vi "EXO RealTime Controls.vi"() -> ()   [LabVIEW 2010]
uses:
  <vilib>/addons/control/pid/pid.llb/PID (DBL).vi
  <vilib>/Utility/error.llb/DialogType.ctl
  <vilib>/Instr/_visa.llb/VISA Configure Serial Port (Instr).vi
  <vilib>/Platform/TimedLoop/XDataNode/XDataNode.xnode
  <vilib>/Platform/TimedLoop/XDataNode/nitl_modes.ctl
  <vilib>/Platform/TimedLoop/XDataNode/XDNodeRunTimeDep.lvlib
  <vilib>/Platform/TimedLoop/XDataNode/wakeup.ctl
  <vilib>/Platform/TimedLoop/XDataNode/timing_clust.ctl
  <vilib>/FieldPoint/Polymorphic Read.llb/FP Read (Boolean -IO).vi
  <vilib>/Utility/file.llb/Write To Spreadsheet File (I64).vi
panel:
  in  "Start Yoyo":bool
  in  "Low dP limit for Yoyo":dbl=-100.0
  in  "High dP limit for Yoyo":dbl=100.0
  in  "Yoyo method while in\nAutomatic?":bool=TRUE
  in  "Yoyo\nMethod\nProp. Valves\nSetting":dbl(slide)=0.04 min=0.0 max=0.075 scale=0.0..0.075
  in  "Automatic Bleed\nWhen in Manual?":bool
  in  "Run All Fridges?":bool
  out "Actual dP Offset (torr)":dbl=100.0
  in  "dP Offset 2 (torr)":dbl
  in  "dP Offset 1 (torr)":dbl
  in  "Bleed 50?":bool
  in  "VX52 real":bool
  in  "Control TC":u16(ring)=37 items=["1", "2", "3", "4", "5", "6", "7", "8", "10", "11", "12", "13", "14", "15", "16", "17", "18", "19", "20", "21", "22", "23", "24", "25", "26", "27", "28", "29", "30", "31", "32", "33", "34", "35", "36", "37", "38", "39", "40"]
  in  "Enter Liquid\nLevel Manually?":bool
  in  "Manual Liquid\nLevel (cm)":dbl
  in  "HFE head disable":bool
  in  "Valves to Open":i32[](array[numeric])=[49, 51, 52, 0, 0, 0]
  out "Actual Pressure\n(psi)":dbl=20.47422134532471
  in  "Cryostat High Liquid\nLevel Alarm (cm)":dbl=300.0 min=0.0
  in  "Cryostat Low Liquid\nLevel Alarm (cm)":dbl=20.0
  in  "Ballast Bottle Low\nLevel Alarm (cm)":dbl min=0.0
  in  "Xenon Heater\nIn Use?":bool
  in  "Ring":u16(ring) items=["Normal Operation", "Vapour Fill Mode", "Pumpout Mode"]
  in  "baud rate 4":u32=9600
  in  "VISA resource name 4":refnum<visa-resource-name>="COM2"
  in  "data bits 4":u16=8 min=5 max=8 step=1
  in  "parity 4":u16(ring) items=["None", "Odd", "Even", "Mark", "Space"]
  in  "stop bits 4":u16(ring)=10 items=["1.0"=10, "1.5"=15, "2.0"=20]
  in  "flow control 4":u16(ring) items=["None"=0, "XON/XOFF"=1, "RTS/CTS"=2, "DTR/DSR"=4]
  in  "Prop Valve\nMult. Factor":dbl=0.04
  in  "V-X9":dbl(slide)=0.042 min=0.0 max=0.075 scale=0.0..0.075
  in  "V-X8":dbl(slide)=0.035 min=0.0 max=0.075 scale=0.0..0.075
  in  "V-X52":bool
  in  "V-X51":bool
  in  "V-X50":bool
  in  "V-X49":bool
  in  "V-X11":bool
  in  "V-X10":bool
  in  "Manual Operation of Valves":bool=TRUE
  in  "Restart all 3 Fridges until setpoint":bool
  in  "baud rate 3":u32=9600
  in  "VISA resource name 3":refnum<visa-resource-name>="COM2"
  in  "data bits 3":u16=8 min=5 max=8 step=1
  in  "parity 3":u16(ring) items=["None", "Odd", "Even", "Mark", "Space"]
  in  "stop bits 3":u16(ring)=10 items=["1.0"=10, "1.5"=15, "2.0"=20]
  in  "flow control 3":u16(ring) items=["None"=0, "XON/XOFF"=1, "RTS/CTS"=2, "DTR/DSR"=4]
  in  "baud rate 2":u32=9600
  in  "VISA resource name 2":refnum<visa-resource-name>="COM3"
  in  "data bits 2":u16=8 min=5 max=8 step=1
  in  "parity 2":u16(ring) items=["None", "Odd", "Even", "Mark", "Space"]
  in  "stop bits 2":u16(ring)=10 items=["1.0"=10, "1.5"=15, "2.0"=20]
  in  "flow control 2":u16(ring) items=["None"=0, "XON/XOFF"=1, "RTS/CTS"=2, "DTR/DSR"=4]
  in  "Condenser \nin Use?":bool=TRUE
  in  "HFE Relief to\nAtmosphere\nThreshold (torr)":dbl=1450.0 min=0.0
  in  "HFE Vapor Fill\nSet Point (torr)":dbl=890.0
  in  "Vapor Fill\nValve \n(HEV17)":bool
  in  "Relief To \nWessington\n(HEV28/18)":bool
  in  "HFE Relief to\nWessington \nThreshold (torr)":dbl=1350.0 min=0.0
  in  "Manual Operation of HFE Valves?":bool
  in  "Ballast Bottle \nHeater in use?":bool=TRUE
  out "Cryostat \nTemp. (K)":dbl=170.03219604492188
  out "Actual":dbl=999.1363027125445
  out "Actual":dbl=167.0546875
  in  "Valve 2 State":bool=TRUE
  in  "Valve 1 State":bool=TRUE
  in  "Manual Operation of Valves":bool
  in  "Heaters In Use?":bool
  in  "Heater Temperature\nHigh Cutoff Limit (K)":dbl=400.0 format="%.2f"
  in  "Cryostat Heater PID Gains":T1={"Proportional gain (Kc)"=1.0, "Integral time (Ti, min)"=0.01, "Derivative time (Td, min)"=0.0} {"Derivative time (Td, min)" format="%.3f"; "Integral time (Ti, min)" format="%.3f"; "Proportional gain (Kc)" format="%.3f"}
  in  "Reinitialize\nHeater PID":bool
  in  "Heater Output \nHigh Limit (Volts)":dbl min=0.0
  in  "Heater Output \nLow Limit (Volts)":dbl min=0.0
  in  "Temperature\nSet Point (K)":dbl=300.0 format="%.2f"
  in  "Folder to Store Data if Monitoring Program fails":string="c:/data/"
  in  "CC Shut-Off\nThreshold (Torr)":dbl=1.0
  in  "CC Soft Threshold\nAlarm (Torr)":dbl=1.0
  in  "TC 1/2 Shut-Off\nThreshold (Torr)":dbl=1.0
  in  "TC 1/2 Soft Threshold\nAlarm (Torr)":dbl=0.05
  in  "flow control":u16(ring) items=["None"=0, "XON/XOFF"=1, "RTS/CTS"=2, "DTR/DSR"=4]
  in  "stop bits":u16(ring)=10 items=["1.0"=10, "1.5"=15, "2.0"=20]
  in  "parity":u16(ring) items=["None", "Odd", "Even", "Mark", "Space"]
  in  "data bits":u16=8 min=5 max=8 step=1
  in  "VISA resource name":refnum<visa-resource-name>="COM1"
  in  "baud rate":u32=9600
  out "Loop Index":i32=402
  in  "Xenon Heater \nOutput \nLow Limit":dbl min=0.0
  in  "Xenon Heater \nOutput \nHigh Limit":dbl min=0.0
  in  "Reinitialize\nXenon Heater PID":bool
  in  "Xenon Heater PID Gains":T1={"Proportional gain (Kc)"=10.0, "Integral time (Ti, min)"=0.1, "Derivative time (Td, min)"=0.0} {"Derivative time (Td, min)" format="%.3f"; "Integral time (Ti, min)" format="%.3f"; "Proportional gain (Kc)" format="%.3f"}
  in  "Max |dP|\nacross purifier":dbl format="%.2f"
  in  "dP across purifier\nset point value":dbl min=0.0
  in  "Recirc. Pump \nOutput \nLow Limit":dbl min=0.0
  in  "Recirc. Pump \nOutput \nHigh Limit":dbl min=0.0
  in  "Reinitialize\nRecirc. Pump PID":bool
  in  "Recirc. Pump PID Gains":T1={"Proportional gain (Kc)"=1.0, "Integral time (Ti, min)"=0.01, "Derivative time (Td, min)"=0.0} {"Derivative time (Td, min)" format="%.3f"; "Integral time (Ti, min)" format="%.3f"; "Proportional gain (Kc)" format="%.3f"}
  in  "Ballast Bottle\nOverpressure (psi)":dbl=26.0 min=0.0
  in  "Reinitialize \nHFE Ballast Bottle\nHeater PID":bool
  in  "HFE Ballast Bottle Heater PID Gains":T1={"Proportional gain (Kc)"=20.0, "Integral time (Ti, min)"=0.0, "Derivative time (Td, min)"=0.0} {"Derivative time (Td, min)" format="%.3f"; "Integral time (Ti, min)" format="%.3f"; "Proportional gain (Kc)" format="%.3f"}
  in  "Low":dbl min=0.0
  in  "High":dbl=60.0 min=0.0
  in  "Set Point":dbl=1000.0 min=0.0
  out "Recirc. Pump output":dbl format="%.2f"
  in  "PT #(After Purifier)":i32
  in  "PT #(Before Purifier)":i32
  in  "High":dbl=60.0 min=0.0
  in  "Low":dbl min=0.0
  in  "Reinitialize\nCondenser PID":bool
  in  "Condenser PID Gains":T1={"Proportional gain (Kc)"=10.0, "Integral time (Ti, min)"=0.2, "Derivative time (Td, min)"=0.0} {"Derivative time (Td, min)" format="%.3f"; "Integral time (Ti, min)" format="%.3f"; "Proportional gain (Kc)" format="%.3f"}
  in  "Set Point":dbl=167.0 min=0.0
  in  "Loop time (sec)":dbl=1.0 min=0.0
  in  "3 Condenser TC's \nVariation Max (K)":dbl=20.0 min=0.0
  in  "Condenser \nOvercool Temp (K)":dbl=165.0 min=0.0
  in  "Cryostat Fridge\nDead Time (s)":dbl=10.0 min=0.0
  in  "Low":dbl=169.95 min=0.0
  in  "High":dbl=170.05 min=0.0
  in  "Inner Cryostat \nTC Variation Max (K)":dbl=1.0 min=0.0
  in  "Inner Cryostat \nOvercool Temp (K)":dbl=160.0 min=0.0
  in  "Feed and Bleed\nDead Time (s)":dbl=1.0 min=0.0
  in  "delta (Dead band)\n(torr)":dbl=15.0 min=0.0
  in  "|dP| Maximum\n(torr)":dbl=250.0 min=0.0
  in  "High Limit\nfor dP Gauge":dbl=1000.0
  in  "Low Limit\nfor dP Gauge":dbl=-1000.0
  in  "Max diff between \ndP from gauge and\ndP from man. (torr)":dbl=50.0 min=0.0
  in  "Inner Cryostat \nOverpress (torr)":dbl=1450.0 min=0.0
  in  "Xe Vessel \nOverpressure (torr)":dbl=1450.0 min=0.0
  in  "2 HFE \nManometers \nMax Var (torr)":dbl=25.0 min=0.0
  in  "2 Xe Manometers \nMax Var (torr)":dbl=25.0 min=0.0
  # "Feed and Bleed Controls"
  # "Inner Cryostat Temperature Controls"
  # "Xenon Heater Controls"
  # "Pumpout Cart"
  # "Control Parameters"
  # "Control Parameters"
  # "Control Parameters"
  # "Control Parameters"
  # "Cryostat Temperature\nSet Points (K)"
  # "Alarm Parameters"
  # "Fridges to Use:"
  # "Alarm Parameters"
  # "Alarm Parameters"
  # "Condenser Temperature Controls"
  # "HFE Ballast Bottle Pressure Controls"
  # "Recirculation Pump Controls"
  # "Cryostat Heaters Controls"
  # "Control Parameters"
  # "Control Parameters"
  # "Control Parameters"
  # "Control Parameters"
  # "Condenser Heater\nLimits (Volts)"
  # "Condenser \nTemperature (K)"
  # "HFE System\nPressure (torr)"
  # "Ballast Bottle\nHeater Limits (Volts)"
  # "Alarm Parameters"
  # "Alarm Parameters"
  # "Alarm Parameters"
  # "Alarm Parameters"
  # "Xenon System Valve States"
  # "HFE System"
  # "Control Parameters"
  # "Operating Mode:"
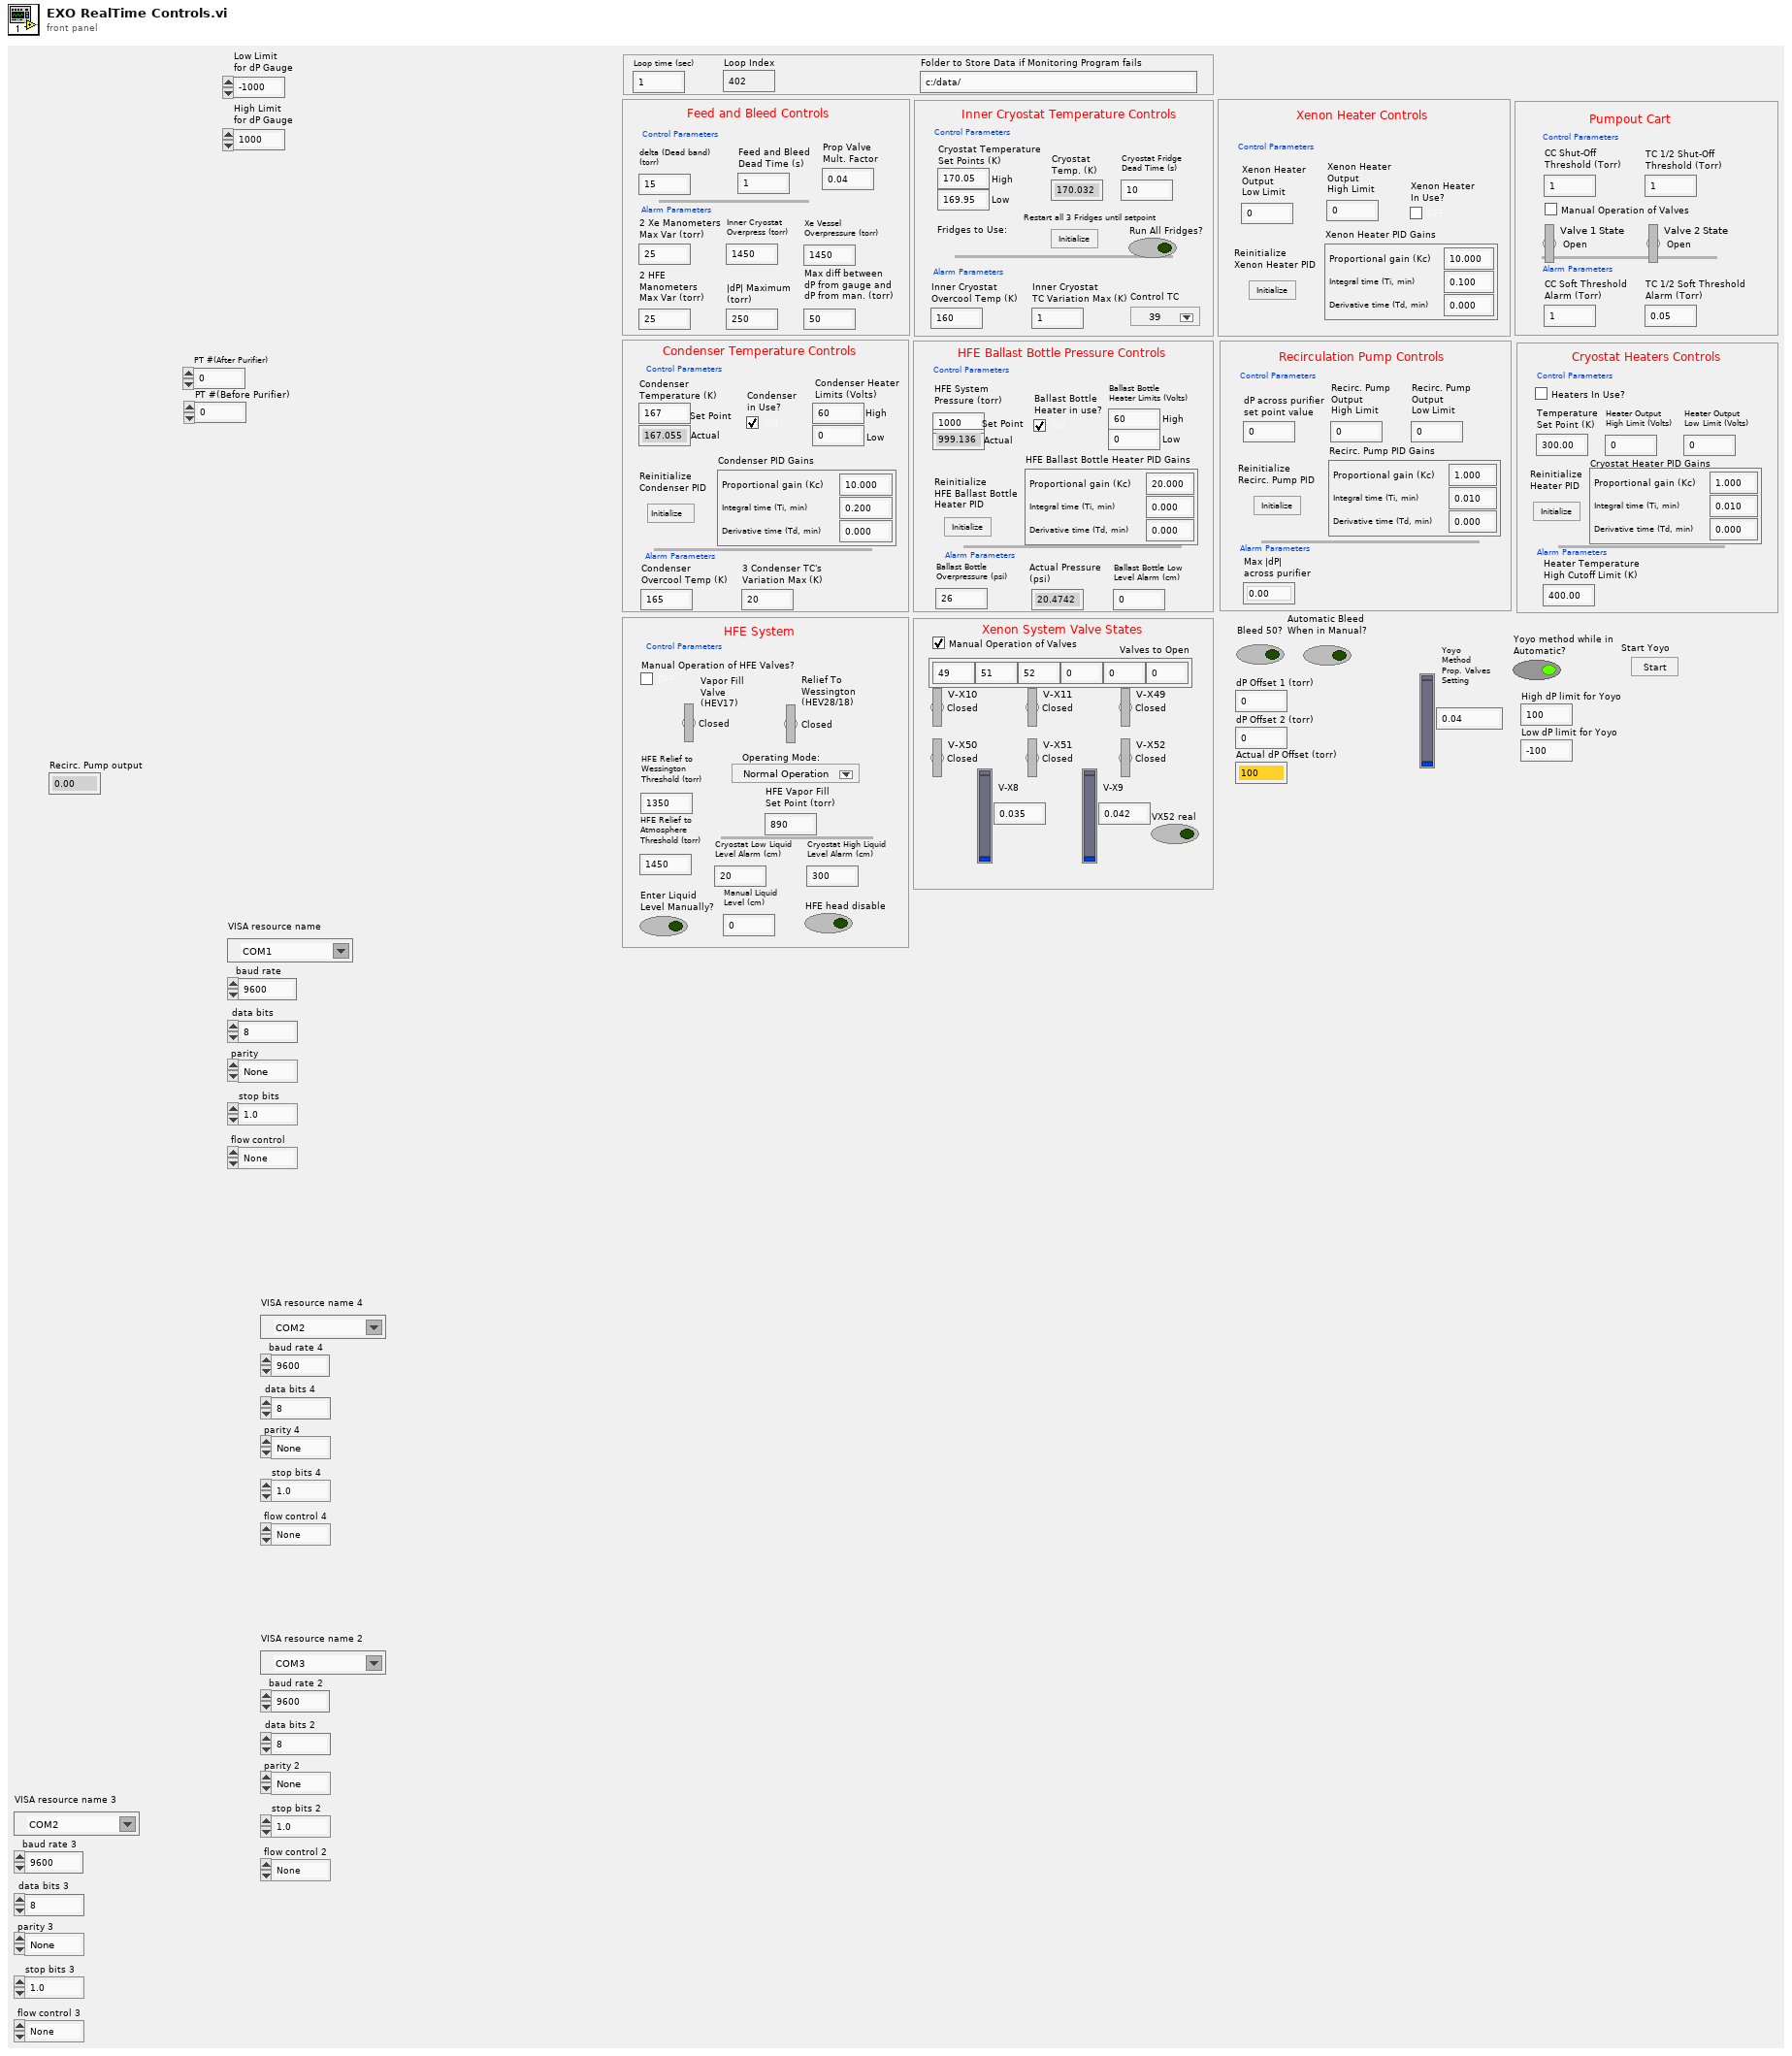
[diagram p1: front panel]
types:
  T1 = cluster{"Proportional gain (Kc)":dbl, "Integral time (Ti, min)":dbl, "Derivative time (Td, min)":dbl}
  T2 = typedef "DialogType.ctl" = u16
  T3 = typedef "XDNodeRunTimeDep.lvlib/nitl_modes.ctl" = enum32{"No Change", "Process missed periods, maintain original phase", "Discard missed periods, maintain original phase", "Process missed periods, ignore original phase", "Discard missed periods, ignore original phase"}
  T4 = typedef "XDNodeRunTimeDep.lvlib/timing_clust.ctl" = cluster{"Expected End [f-1]":u64, "Actual End [f-1]":u64, "Finished Late? [f-1]":bool, "Expected End [i-1]":u64, "Actual End [i-1]":u64, "Finished Late? [i-1]":bool, "Expected Start [i]":u64, "Actual Start [i]":u64, "Expected Start [f]":u64, "Actual Start [f]":u64, "Source Name":string, "Structure Name":string, "Period":i64, "Deadline":i64, "Offset":i64, "Start":i64, "Priority":i32, "Timeout":i32, "Mode":T3, "Wakeup Reason":T5, "Error":errorcluster, "Source Type":string, "Secondary Source Type":string, "Global End Time":u64, "Global Start Time":u64, "Frame Duration":u64, "Iteration Duration":u64, "Assigned CPU":i32, "I/O Scan Engine Mode":u32}
  T5 = typedef "XDNodeRunTimeDep.lvlib/wakeup.ctl" = enum32{"Normal", "Aborted", "Asynchronous wakeup", "Timing source error", "Timed loop error", "Timeout"}
  T6 = cluster{"Heater Output \nLow Limit (Volts)":dbl, "Heater Output \nLow Limit (Volts)":dbl}
  T7 = cluster{"Xenon Heater \nOutput \nLow Limit":dbl, "Xenon Heater \nOutput \nLow Limit":dbl}
  T8 = cluster{"Recirc. Pump \nOutput \nLow Limit":dbl, "Recirc. Pump \nOutput \nLow Limit":dbl}
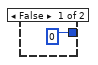
[diagram p2: hidden frame]
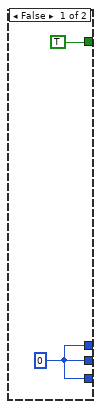
[diagram p3: hidden frame]
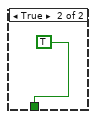
[diagram p10: hidden frame]
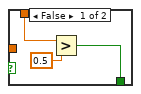
[diagram p11: hidden frame]
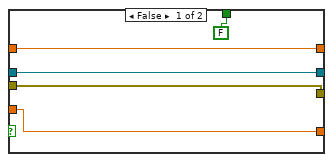
[diagram p12: hidden frame]
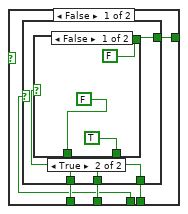
[diagram p13: hidden frame]
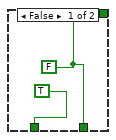
[diagram p14: hidden frame]
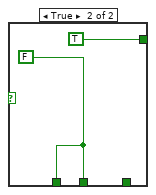
[diagram p15: hidden frame]
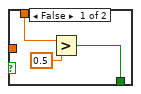
[diagram p16: hidden frame]
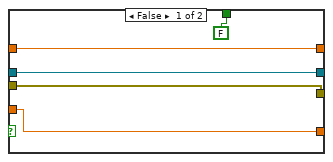
[diagram p17: hidden frame]
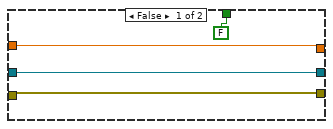
[diagram p18: hidden frame]
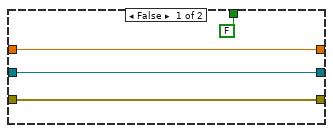
[diagram p19: hidden frame]
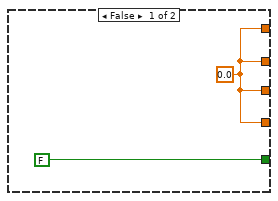
[diagram p20: hidden frame]
diagram:
  w6 = T2 0 items=["no dialog", "OK message", "continue or stop message", "OK message + warnings", "continue/stop + warnings"] ("type of dialog (OK msg:1)")
  w8 = 0.0 ("index")
  w18 = T2 0 items=["no dialog", "OK message", "continue or stop message", "OK message + warnings", "continue/stop + warnings"] ("type of dialog (OK msg:1)")
  w21 = FALSE  # Enable Termination Char (T)
  w22 = u32 10000  # timeout (10sec)
  w35 = T2 0 items=["no dialog", "OK message", "continue or stop message", "OK message + warnings", "continue/stop + warnings"] ("type of dialog (OK msg:1)")
  w36 = FALSE  # Enable Termination Char (T)
  w37 = u32 10000  # timeout (10sec)
  w46 = T2 0 items=["no dialog", "OK message", "continue or stop message", "OK message + warnings", "continue/stop + warnings"] ("type of dialog (OK msg:1)")
  w57 = FALSE  # Enable Termination Char (T)
  w56 = u32 10000  # timeout (10sec)
  w65 = T2 0 items=["no dialog", "OK message", "continue or stop message", "OK message + warnings", "continue/stop + warnings"] ("type of dialog (OK msg:1)")
  w97 = T2 0 items=["no dialog", "OK message", "continue or stop message", "OK message + warnings", "continue/stop + warnings"] ("type of dialog (OK msg:1)")
  w104 = T2 0 items=["no dialog", "OK message", "continue or stop message", "OK message + warnings", "continue/stop + warnings"] ("type of dialog (OK msg:1)")
  w120 = T2 0 items=["no dialog", "OK message", "continue or stop message", "OK message + warnings", "continue/stop + warnings"] ("type of dialog (OK msg:1)")
  w123 = FALSE  # Enable Termination Char (T)
  w124 = u32 10000  # timeout (10sec)
  # "Close RS232 Connection"
  # "Close RS232 Connection"
  # "Close RS232 Connection"
  # "Close RS232 Connection"
  # "Initialization of RS232 Port\non the Controler"
  # "Close RS232 Connection"
  # "Initialize\nDouble Array"
  # "Initialize\nBoolean Array"
  # "Initialize\nBoolean Array"
  # "Initialize\nDouble Array"
  # "Initialize\nDouble Array"
  # "Initialize\nError Array"
  # "Initialize\nBoolean Array"
  # "Initialize\nData Array"
  # "Close RS232 Connection"
  # "Close RS232 Connection"
  # "Recording Data"
  # "Close RS232 Connection"
  # "Initialization of RS232 Port\non the Controler"
  n1 = call-poly "VISA Configure Serial Port"("VISA resource name"="VISA resource name 3", "timeout (10sec)"=w37, "Enable Termination\nChar (T)"=w36, "baud rate (9600)"="baud rate 3", "data bits (8)"="data bits 3", "parity (0:none)"="parity 3", "stop bits (10: 1 bit)"="stop bits 3", "flow control (0:none)"="flow control 3") -> ("VISA resource name out"=w33:refnum<visa-resource-name>, "error out"=w32:errorcluster)  [unwired: 6 in]
  n2 = Multiply(x=1000 ("y"), y="Loop time (sec)") -> (x*y=w108:dbl)
  n3 = Initialize Array(0.0 ("element"), 200 ("dimension size")) -> (w85:dbl[])
  n4 = call-poly "VISA Configure Serial Port"("VISA resource name"="VISA resource name", "timeout (10sec)"=w124, "Enable Termination\nChar (T)"=w123, "baud rate (9600)"="baud rate", "data bits (8)"="data bits", "parity (0:none)"="parity", "stop bits (10: 1 bit)"="stop bits", "flow control (0:none)"="flow control") -> ("VISA resource name out"=w122:refnum<visa-resource-name>, "error out"=w121:errorcluster)  [unwired: 6 in]
  n5 = call-poly "VISA Configure Serial Port"("VISA resource name"="VISA resource name 4", "timeout (10sec)"=w22, "Enable Termination\nChar (T)"=w21, "baud rate (9600)"="baud rate 4", "data bits (8)"="data bits 4", "parity (0:none)"="parity 4", "stop bits (10: 1 bit)"="stop bits 4", "flow control (0:none)"="flow control 4") -> ("VISA resource name out"=w20:refnum<visa-resource-name>, "error out"=w19:errorcluster)  [unwired: 6 in]
  n6 = call-poly "VISA Configure Serial Port"("VISA resource name"="VISA resource name 2", "timeout (10sec)"=w56, "Enable Termination\nChar (T)"=w57, "baud rate (9600)"="baud rate 2", "data bits (8)"="data bits 2", "parity (0:none)"="parity 2", "stop bits (10: 1 bit)"="stop bits 2", "flow control (0:none)"="flow control 2") -> ("VISA resource name out"=w49:refnum<visa-resource-name>, "error out"=w48:errorcluster)  [unwired: 6 in]
  n7 = node-c288(w108, nitl_modes."Discard missed periods, ignore original phase" ("Mode")) -> (w116:T4)  [unwired: 8 in]
  n8 = call-poly "VISA Configure Serial Port"("VISA resource name"=refnum<visa-resource-name> "COM4" ("VISA resource name 2")) -> ("VISA resource name out"=w106:refnum<visa-resource-name>, "error out"=w105:errorcluster)  [unwired: 13 in]
  n9 = call-poly "VISA Configure Serial Port"("VISA resource name"=refnum<visa-resource-name> "COM4" ("VISA resource name 2")) -> ("VISA resource name out"=w100:refnum<visa-resource-name>, "error out"=w99:errorcluster)  [unwired: 13 in]
  n10 = call-poly "VISA Configure Serial Port"("VISA resource name"=refnum<visa-resource-name> "COM1" ("VISA resource name 2")) -> ("VISA resource name out"=w67:refnum<visa-resource-name>, "error out"=w66:errorcluster)  [unwired: 13 in]
  n11 = call-poly "VISA Configure Serial Port"("VISA resource name"=refnum<visa-resource-name> "COM3" ("VISA resource name 2")) -> ("VISA resource name out"=w10:refnum<visa-resource-name>, "error out"=w9:errorcluster)  [unwired: 13 in]
  n12 = Initialize Array(TRUE, 4 ("dimension size")) -> (w73:bool[])
  n13 = Initialize Array(0.0, 3 ("dimension size")) -> (w79:dbl[])
  n14 = Initialize Array(TRUE, 3 ("dimension size")) -> (w76:bool[])
  n15 = Initialize Array(0.0, 2 ("dimension size")) -> (w58:dbl[])
  n16 = Initialize Array("", 5 ("dimension size")) -> (w13:string[])
  n17 = Initialize Array(FALSE, 200 ("dimension size")) -> (w88:bool[])
  n18 = Initialize Array(0.0, 8 ("dimension size")) -> (w82:dbl[])
  n19 = Initialize Array("12345", 6 ("dimension size")) -> (w69:string[])
  n20 = Initialize Array(0.0 ("element"), 250 ("dimension size")) -> (w91:dbl[])
  n21 = timed-loop {
    shift-right: [w282] -> _
    shift-left: 0 ("index") -> [w288]
    shift-right: [w281] -> _
    shift-left: -2 ("index") -> [w287]
    shift-right: [w283] -> _
    shift-left: 0 ("index") -> [w286]
    shift-right: [w284] -> _
    shift-left: -2 ("index of element") -> [w285]
    tunnel: "Loop time (sec)" -> [w272]
    tunnel: w122 -> [w280]
    tunnel: w121 -> [w279]
    tunnel: [w278] -> w118
    tunnel: [w277] -> w117
    shift-right: [w274] -> _
    shift-left: _ -> [w276]
    shift-right: [w273] -> _
    shift-left: _ -> [w275]
    timing: w116 -> [_]
    timing-out: [_] -> w115
    tunnel: w106 -> [w256]
    tunnel: w105 -> [w255]
    tunnel: [w252] -> w102
    tunnel: [w251] -> w101
    tunnel: w100 -> [w250]
    tunnel: w99 -> [w249]
    tunnel: [w246] -> w96
    tunnel: [w245] -> w95
    shift-right: [w241] -> _
    shift-left: _ -> [w238]
    shift-right: [w240] -> _
    shift-left: _ -> [w239]
    tunnel: w91 -> [w233]
    tunnel: w88 -> [w232]
    tunnel: w85 -> [w230]
    tunnel: w82 -> [w228]
    tunnel: w79 -> [w226]
    tunnel: w76 -> [w224]
    tunnel: w73 -> [w222]
    tunnel: "12345678901234567890" -> [w220]
    tunnel: w69 -> [w219]
    tunnel: w67 -> [w217]
    tunnel: w66 -> [w216]
    tunnel: [w215] -> w63
    tunnel: [w214] -> w62
    shift-right: [w212] -> _
    shift-left: _ -> [w213]
    shift-right: [w204] -> _
    shift-left: _ -> [w205]
    shift-right: [w202] -> _
    shift-left: _ -> [w201]
    tunnel: w58 -> [w197]
    tunnel: w49 -> [w196]
    tunnel: w48 -> [w195]
    tunnel: [w192] -> w45
    tunnel: [w191] -> w44
    tunnel: w33 -> [w188]
    tunnel: w32 -> [w187]
    tunnel: [w182] -> w31
    tunnel: [w181] -> w30
    shift-right: [w180] -> _
    shift-left: 1.0 -> [w178]
    shift-right: [w176] -> _
    shift-left: _ -> [w175]
    tunnel: w20 -> [w173]
    tunnel: w19 -> [w172]
    tunnel: [w169] -> w16
    tunnel: [w168] -> w15
    tunnel: w13 -> [w167]
    shift-right: [w165] -> _
    shift-left: _ -> [w163]
    shift-right: [w164] -> _
    shift-left: _ -> [w161]
    tunnel: w10 -> [w159]
    tunnel: w9 -> [w158]
    shift-right: [w148] -> _
    shift-left: w8 -> [w157]
    shift-right: [w150] -> _
    shift-left: w8 -> [w156]
    tunnel: [w155] -> w5
    tunnel: [w154] -> w4
    shift-right: [w142] -> _
    shift-left: _ -> [w143]
    shift-right: [w137] -> _
    shift-left: 0.0 -> [w139]
    shift-right: [w134] -> _
    shift-left: 0 ("dimension size") -> [w135]
    i -> [w237]
    stop <- FALSE ("stop") stop-if-true
    n22 = node-c288() -> ()  [unwired: 1 in, 1 out]
    n23 = Equal To 0?(x=w178) -> (x = 0?=w179:bool)
    n24 = flat-sequence {
      tunnel: w272 -> [w594]
      tunnel: w275 -> [w564]
      tunnel: w276 -> [w565]
      tunnel: w279 -> [w595]
      tunnel: w280 -> [w596]
      tunnel: w285 -> [w597]
      tunnel: w286 -> [w598]
      tunnel: w287 -> [w599]
      tunnel: w288 -> [w600]
      tunnel: [w600] -> w270
      tunnel: [w599] -> w269
      tunnel: [w598] -> w268
      tunnel: [w597] -> w267
      tunnel: [w596] -> w266
      tunnel: [w595] -> w265
      tunnel: [w594] -> w264
      tunnel: [w371] -> w263
      tunnel: [w370] -> w262
      tunnel: [w305] -> w261
      tunnel: [w553] -> w260
      tunnel: [w552] -> w259
      tunnel: [w550] -> w258
      tunnel: [w549] -> w257
      tunnel: w256 -> [w548]
      tunnel: w255 -> [w547]
      tunnel: [w546] -> w254
      tunnel: [w545] -> w253
      tunnel: w250 -> [w544]
      tunnel: w249 -> [w543]
      tunnel: [w542] -> w248
      tunnel: [w541] -> w247
      tunnel: [w539] -> w244
      tunnel: [w537] -> w243
      tunnel: [w314] -> w242
      tunnel: w239 -> [w535]
      tunnel: w238 -> [w534]
      tunnel: w237 -> [w532]
      tunnel: ["Heaters In Use?"] -> w236
      tunnel: [w499] -> w235
      tunnel: [w498] -> w234
      tunnel: w233 -> [w498]
      tunnel: w232 -> [w436]
      tunnel: [w497] -> w231
      tunnel: w230 -> [w496]
      tunnel: [w494] -> w229
      tunnel: w228 -> [w473]
      tunnel: [w473] -> w227
      tunnel: w226 -> [w472]
      tunnel: [w472] -> w225
      tunnel: w224 -> [w471]
      tunnel: [w471] -> w223
      tunnel: w222 -> [w470]
      tunnel: [w470] -> w221
      tunnel: w219 -> [w469]
      tunnel: [w469] -> w218
      tunnel: w217 -> [w468]
      tunnel: w216 -> [w467]
      tunnel: w213 -> [w461]
      tunnel: [w460] -> w211
      tunnel: ["Ballast Bottle \nHeater in use?"] -> w210
      tunnel: [w314] -> w209
      tunnel: [w459] -> w208
      tunnel: [w458] -> w207
      tunnel: [w457] -> w206
      tunnel: w205 -> [w456]
      tunnel: [w446] -> w203
      tunnel: w201 -> [w455]
      tunnel: [w438] -> w200
      tunnel: [w437] -> w199
      tunnel: [w424] -> w198
      tunnel: w197 -> [w424]
      tunnel: w196 -> [w421]
      tunnel: w195 -> [w420]
      tunnel: [w419] -> w194
      tunnel: [w418] -> w193
      tunnel: [w402] -> w190
      tunnel: [w401] -> w189
      tunnel: w188 -> [w383]
      tunnel: w187 -> [w382]
      tunnel: [w381] -> w186
      tunnel: [w380] -> w185
      tunnel: [w379] -> w184
      tunnel: [w378] -> w183
      tunnel: w179 -> [w293]
      tunnel: w178 -> [w369]
      tunnel: [w369] -> w177
      tunnel: w175 -> [w368]
      tunnel: [w368] -> w174
      tunnel: w173 -> [w367]
      tunnel: w172 -> [w366]
      tunnel: [w362] -> w171
      tunnel: [w361] -> w170
      tunnel: w167 -> [w353]
      tunnel: [w343] -> w166
      tunnel: w163 -> [w342]
      tunnel: [w342] -> w162
      tunnel: w161 -> [w341]
      tunnel: [w341] -> w160
      tunnel: w159 -> [w322]
      tunnel: w158 -> [w321]
      tunnel: w157 -> [w320]
      tunnel: w156 -> [w319]
      tunnel: [w318] -> w153
      tunnel: [w317] -> w152
      tunnel: [w316] -> w151
      tunnel: [w315] -> w149
      tunnel: [w314] -> w147
      tunnel: [w313] -> w146
      tunnel: [w312] -> w145
      tunnel: [w311] -> w144
      tunnel: w143 -> [w308]
      tunnel: [w307] -> w141
      tunnel: ["Xenon Heater\nIn Use?"] -> w140
      tunnel: w139 -> [w295]
      tunnel: [w295] -> w138
      tunnel: w135 -> [w291]
      tunnel: [w291] -> w136
      tunnel: [w1763] -> w284
      tunnel: [w1762] -> w283
      tunnel: [w1761] -> w282
      tunnel: [w1760] -> w281
      tunnel: [w1749] -> w278
      tunnel: [w1748] -> w277
      tunnel: [w1096] -> w274
      tunnel: [w1094] -> w273
      tunnel: w270 -> [w1798]
      tunnel: w269 -> [w1778]
      tunnel: w268 -> [w1773]
      tunnel: w267 -> [w1769]
      tunnel: w266 -> [w1752]
      tunnel: w265 -> [w1751]
      tunnel: w264 -> [w1372]
      tunnel: w263 -> [w1697]
      tunnel: w262 -> [w1695]
      tunnel: w261 -> [w1694]
      tunnel: w260 -> [w1316]
      tunnel: w259 -> [w1682]
      tunnel: w258 -> [w1595]
      tunnel: w257 -> [w1596]
      tunnel: w254 -> [w1681]
      tunnel: w253 -> [w1680]
      tunnel: [w1679] -> w252
      tunnel: [w1678] -> w251
      tunnel: w248 -> [w1673]
      tunnel: w247 -> [w1672]
      tunnel: [w1671] -> w246
      tunnel: [w1670] -> w245
      tunnel: w244 -> [w1420]
      tunnel: w243 -> [w1614]
      tunnel: w242 -> [w1669]
      tunnel: [w1420] -> w241
      tunnel: [w1614] -> w240
      tunnel: w236 -> [w1603]
      tunnel: w235 -> [w1570]
      tunnel: w234 -> [w1569]
      tunnel: w231 -> [w1559]
      tunnel: w229 -> [w1555]
      tunnel: w227 -> [w1470]
      tunnel: w225 -> [w1465]
      tunnel: w223 -> [w1457]
      tunnel: w221 -> [w1447]
      tunnel: w220 -> [w829]
      tunnel: w218 -> [w1423]
      tunnel: [w1383] -> w215
      tunnel: [w1382] -> w214
      tunnel: [w1130] -> w212
      tunnel: w211 -> [w1130]
      tunnel: w210 -> [w1375]
      tunnel: w209 -> [w863]
      tunnel: w208 -> [w1365]
      tunnel: w207 -> [w1361]
      tunnel: w206 -> [w1360]
      tunnel: [w1351] -> w204
      tunnel: w203 -> [w1351]
      tunnel: [w1349] -> w202
      tunnel: w200 -> [w1346]
      tunnel: w199 -> [w1345]
      tunnel: w198 -> [w1289]
      tunnel: w194 -> [w1261]
      tunnel: w193 -> [w1262]
      tunnel: [w1262] -> w192
      tunnel: [w1261] -> w191
      tunnel: w190 -> [w1259]
      tunnel: w189 -> [w1257]
      tunnel: w186 -> [w1255]
      tunnel: w185 -> [w1253]
      tunnel: w184 -> [w1252]
      tunnel: w183 -> [w1251]
      tunnel: [w1252] -> w182
      tunnel: [w1251] -> w181
      tunnel: [w1207] -> w180
      tunnel: w177 -> [w1209]
      tunnel: [w807] -> w176
      tunnel: w174 -> [w1155]
      tunnel: w171 -> [w1145]
      tunnel: w170 -> [w1144]
      tunnel: [w1143] -> w169
      tunnel: [w1142] -> w168
      tunnel: w166 -> [w1139]
      tunnel: [w809] -> w165
      tunnel: [w864] -> w164
      tunnel: w162 -> [w1111]
      tunnel: w160 -> [w1110]
      tunnel: [w1073] -> w155
      tunnel: [w1072] -> w154
      tunnel: w153 -> [w1071]
      tunnel: w152 -> [w1070]
      tunnel: w151 -> [w1069]
      tunnel: [w1069] -> w150
      tunnel: w149 -> [w1037]
      tunnel: [w1037] -> w148
      tunnel: w147 -> [w1068]
      tunnel: w146 -> [w1064]
      tunnel: w145 -> [w1063]
      tunnel: w144 -> [w1062]
      tunnel: [w847] -> w142
      tunnel: w141 -> [w1035]
      tunnel: w140 -> [w845]
      tunnel: w138 -> [w823]
      tunnel: [w780] -> w137
      tunnel: w136 -> [w771]
      tunnel: [w787] -> w134
      frame #0 {
        (unwired) 1 ("index")
        w354 = 9 ("length (rest)")
        w373 = refnum<k21> "FieldPoint\\MPR2\\Digital Voltage Input Module 2\\All"  # FieldPoint IO Point
        w375 = refnum<k21> "FieldPoint\\MET1\\cFP-DI-330 @4\\All"  # FieldPoint IO Point
        w377 = refnum<k21> "FieldPoint\\MET1\\cFP-DI-330 @3\\All"  # FieldPoint IO Point
        w428 = refnum<k21> "FieldPoint\\MPR2\\Digital Voltage Input Module 3\\All"  # FieldPoint IO Point
        w432 = refnum<k21> "FieldPoint\\MPR1\\Digital Voltage Input Module 1\\All"  # FieldPoint IO Point
        # "Scale L Data"
        # "Scale R Data"
        # "Read Info From Power Supply 2"
        # "Read Info From Power Supply 1"
        # "PC #10"
        # "PC #9"
        # "PC #5"
        # "PC #4"
        # "Pumpout\nCart Status\n(DI)"
        # "Polycold\n3 Status\nData"
        # "Polycold\n1/2 Status\nData"
        n25 = call <vilib>:"FP Read (Boolean Array -IO).vi"("FieldPoint IO Point In"=w375) -> ("value"=w374:bool[])  [unwired: 11 in, 3 out]
        n26 = call <vilib>:"FP Read (Boolean Array -IO).vi"("FieldPoint IO Point In"=w377) -> ("value"=w376:bool[])  [unwired: 11 in, 3 out]
        n27 = Quotient & Remainder(x=w532, y=2) -> (x-y*floor(x/y)=w531:i32)  [unwired: 1 out]
        n28 = call <vilib>:"FP Read (Boolean Array -IO).vi"("FieldPoint IO Point In"=w428) -> ("value"=w427:bool[])  [unwired: 11 in, 3 out]
        n29 = call <vilib>:"FP Read (Boolean Array -IO).vi"("FieldPoint IO Point In"=w373) -> ("value"=w372:bool[])  [unwired: 11 in, 3 out]
        n30 = call <vilib>:"FP Read (Boolean Array -IO).vi"("FieldPoint IO Point In"=w432) -> ("value"=w431:bool[])  [unwired: 11 in, 3 out]
        n31 = Equal To 0?(x=w531) -> (x = 0?=w314:bool)
        n32 = property class="Instr"(reference=w421, error in=w420) -> (reference out=w423:refnum<visa-resource-name>, error out=w422:errorcluster, "Serial Settings:Number of Bytes at Serial Port"=w414:u32)
        n33 = Index Array(array=w376, index #1=0 ("index"), index #2=1 ("index"), index #3=2 ("index"), index #4=3 ("index"), index #5=4 ("index"), index #6=5 ("index"), index #7=6 ("index"), index #8=7 ("index")) -> (element #1=w301:bool, element #2=w585:bool, element #3=w303:bool, element #4=w302:bool, element #5=w298:bool, element #6=w584:bool, element #7=w299:bool, element #8=w300:bool)
        n34 = Index Array(array=w374, index #1=0 ("index"), index #2=1 ("index"), index #3=2 ("index"), index #4=3 ("index"), index #5=4 ("index"), index #6=5 ("index"), index #7=6 ("index"), index #8=7 ("index")) -> (element #1=w572:bool, element #2=w573:bool, element #3=w574:bool, element #4=w575:bool)  [unwired: 4 out]
        n35 = property class="Instr"(reference=w383, error in=w382) -> (reference out=w384:refnum<visa-resource-name>, error out=w385:errorcluster, "Serial Settings:Number of Bytes at Serial Port"=w389:u32)
        n36 = Array Subset(array=w431, index=6) -> (w429:bool[])  [unwired: 1 in]
        n37 = case shown="False" "Run All Fridges?" {
          tunnel: [w601 TRUE] -> w294
          tunnel: w293 -> [w601 _]
          frame False {
          }
          frame True {
          }
        }
        n38 = case shown="True" w314 {
          tunnel: w467 -> [w662 w671]
          tunnel: [w662 w675] -> w457
          tunnel: [w661 w674] -> w458
          tunnel: w468 -> [w661 w673]
          tunnel: [w659 w668] -> w445
          tunnel: [FALSE w666] -> w462
          tunnel: w461 -> [w659 _]
          tunnel: [w658 w663] -> w446
          tunnel: w456 -> [w658 _]
          frame False {
          }
          frame True {
            n39 = property class="Instr"(reference=w673, error in=w671) -> (reference out=w672:refnum<visa-resource-name>, error out=w670:errorcluster, "Serial Settings:Number of Bytes at Serial Port"=w667:u32)
            n40 = Equal To 0?(x=w667) -> (x = 0?=w666:bool)
            n41 = VISA Read(VISA resource name=w672, byte count=w667, error in (no error)=w670) -> (VISA resource name out=w674:refnum<visa-resource-name>, read buffer=w665:string, error out=w675:errorcluster)  [unwired: 1 out]
            n42 = Fract/Exp String To Number(string=w665, offset=5) -> (number=w668:dbl)  [unwired: 2 in, 1 out]
            n43 = Fract/Exp String To Number(string=w665, offset=19) -> (number=w663:dbl)  [unwired: 2 in, 1 out]
          }
        }
        n44 = case shown="True" w314 {
          tunnel: w321 -> [w617 w626]
          tunnel: [w617 w630] -> w317
          tunnel: [w616 w629] -> w318
          tunnel: w322 -> [w616 w628]
          tunnel: [w614 w623] -> w335
          tunnel: [FALSE w621] -> w327
          tunnel: w320 -> [w614 _]
          tunnel: [w613 w618] -> w316
          tunnel: w319 -> [w613 _]
          frame False {
          }
          frame True {
            n45 = property class="Instr"(reference=w628, error in=w626) -> (reference out=w627:refnum<visa-resource-name>, error out=w625:errorcluster, "Serial Settings:Number of Bytes at Serial Port"=w622:u32)
            n46 = Equal To 0?(x=w622) -> (x = 0?=w621:bool)
            n47 = VISA Read(VISA resource name=w627, byte count=w622, error in (no error)=w625) -> (VISA resource name out=w629:refnum<visa-resource-name>, read buffer=w620:string, error out=w630:errorcluster)  [unwired: 1 out]
            n48 = Fract/Exp String To Number(string=w620, offset=5) -> (number=w623:dbl)  [unwired: 2 in, 1 out]
            n49 = Fract/Exp String To Number(string=w620, offset=19) -> (number=w618:dbl)  [unwired: 2 in, 1 out]
          }
        }
        n50 = Compound Arithmetic op=AND(w301, w303, w302) -> (w304:bool)
        n51 = case shown="True" w314 {
          tunnel: w547 -> [w694 w701]
          tunnel: [w694 w705] -> w545
          tunnel: [w693 w704] -> w546
          tunnel: w548 -> [w693 w703]
          tunnel: [w692 w697] -> w540
          tunnel: [FALSE w696] -> w530
          tunnel: w534 -> [w692 _]
          frame False {
          }
          frame True {
            n52 = property class="Instr"(reference=w703, error in=w701) -> (reference out=w702:refnum<visa-resource-name>, error out=w700:errorcluster, "Serial Settings:Number of Bytes at Serial Port"=w695:u32)
            n53 = Equal To 0?(x=w695) -> (x = 0?=w696:bool)
            n54 = VISA Read(VISA resource name=w702, byte count=w695, error in (no error)=w700) -> (VISA resource name out=w704:refnum<visa-resource-name>, read buffer=w699:string, error out=w705:errorcluster)  [unwired: 1 out]
            n55 = Fract/Exp String To Number(string=w699, offset=5) -> (number=w697:dbl)  [unwired: 2 in, 1 out]
          }
        }
        n56 = Index Array(array=w372, index #1=0 ("index"), index #2=1 ("index"), index #3=2 ("index"), index #4=3 ("index"), index #5=4 ("index"), index #6=5 ("index")) -> (element #1=w556:bool, element #2=w557:bool, element #3=w555:bool, element #4=w554:bool, element #5=w553:bool, element #6=w552:bool)
        n57 = Compound Arithmetic op=AND(w298, w299, w300) -> (w297:bool)
        n58 = case shown="True" w294 {
          tunnel: [w635 w647] -> w371
          tunnel: [w634 w647] -> w370
          tunnel: [w633 w647] -> w305
          tunnel: w304 -> [w632 _]
          tunnel: w297 -> [w631 _]
          frame False {
            n59 = case shown="False" w632 {
              tunnel: [w637 TRUE] -> w635
              tunnel: [w639 w645] -> w634
              tunnel: [w638 w645] -> w633
              tunnel: w631 -> [w636 _]
              frame False {
                n60 = case shown="True" w636 {
                  tunnel: [w641 TRUE] -> w639
                  tunnel: [TRUE FALSE] -> w638
                  tunnel: [w641 FALSE] -> w637
                  frame False {
                    w641 = FALSE
                  }
                  frame True {
                  }
                }
              }
              frame True {
                w645 = FALSE
              }
            }
          }
          frame True {
            w647 = TRUE
          }
        }
        n61 = case shown="True" w314 {
          tunnel: w543 -> [w679 w686]
          tunnel: [w679 w690] -> w541
          tunnel: [w678 w689] -> w542
          tunnel: w544 -> [w678 w688]
          tunnel: [w677 w682] -> w536
          tunnel: [FALSE w680] -> w529
          tunnel: w535 -> [w677 _]
          frame False {
          }
          frame True {
            n62 = property class="Instr"(reference=w688, error in=w686) -> (reference out=w687:refnum<visa-resource-name>, error out=w685:errorcluster, "Serial Settings:Number of Bytes at Serial Port"=w681:u32)
            n63 = Equal To 0?(x=w681) -> (x = 0?=w680:bool)
            n64 = VISA Read(VISA resource name=w687, byte count=w681, error in (no error)=w685) -> (VISA resource name out=w689:refnum<visa-resource-name>, read buffer=w683:string, error out=w690:errorcluster)  [unwired: 1 out]
            n65 = Fract/Exp String To Number(string=w683, offset=5) -> (number=w682:dbl)  [unwired: 2 in, 1 out]
          }
        }
        n66 = property class="Instr"(reference=w367, error in=w366) -> (reference out=w365:refnum<visa-resource-name>, error out=w364:errorcluster, "Serial Settings:Number of Bytes at Serial Port"=w363:u32)
        n67 = case shown="True" w305 {
          tunnel: w575 -> [_ w708]
          tunnel: w574 -> [_ w709]
          tunnel: w573 -> [_ w710]
          tunnel: w572 -> [_ w711]
          tunnel: [FALSE ("Polycold 1 Status") w710] -> w516
          tunnel: [w706 w715] -> w507
          tunnel: [w706 w714] -> w506
          tunnel: [w706 w713] -> w505
          tunnel: [w706 w712] -> w504
          frame False {
            w706 = 0.0 ("index")
          }
          frame True {
            n68 = shared-variable "MPR1\\Real-Time Library.lvlib\\Polycold 3 Status"() -> (w724:bool)  [unwired: 1 in, 1 out]
            n69 = Select(t=0.0 ("index"), s=w709, f=14.0 ("index")) -> (s? t:f=w715:dbl)
            n70 = Select(t=0.0 ("index"), s=w711, f=16.0 ("index")) -> (s? t:f=w713:dbl)
            n71 = Equal?(x=w710, y=w724) -> (x = y?=w725:bool)
            n72 = Select(t=0.0 ("index"), s=w708, f=15.0 ("index")) -> (s? t:f=w714:dbl)
            n73 = Select(t=0.0 ("index"), s=w725, f=17.0 ("index")) -> (s? t:f=w712:dbl)
          }
        }
        n74 = case shown="True" w371 {
          tunnel: w301 -> [_ w751]
          tunnel: w585 -> [_ w750]
          tunnel: w303 -> [_ w749]
          tunnel: w302 -> [_ w748]
          tunnel: [FALSE ("Polycold 1 Status") w750] -> w518
          tunnel: [w746 w755] -> w515
          tunnel: [w746 w754] -> w514
          tunnel: [w746 w753] -> w513
          tunnel: [w746 w752] -> w512
          frame False {
            w746 = 0.0 ("index")
          }
          frame True {
            # "8"
            # "6"
            n75 = shared-variable "MPR1\\Real-Time Library.lvlib\\Polycold 1 Status"() -> (w764:bool)  [unwired: 1 in, 1 out]
            n76 = Select(t=0.0 ("index"), s=w749, f=6.0 ("index")) -> (s? t:f=w755:dbl)
            n77 = Select(t=0.0 ("index"), s=w751, f=8.0 ("index")) -> (s? t:f=w753:dbl)
            n78 = Select(t=0.0 ("index"), s=w748, f=7.0 ("index")) -> (s? t:f=w754:dbl)
            n79 = Equal?(x=w764, y=w750) -> (x = y?=w765:bool)
            n80 = Select(t=0.0 ("index"), s=w765, f=9.0 ("index")) -> (s? t:f=w752:dbl)
          }
        }
        n81 = case shown="True" w370 {
          tunnel: w298 -> [_ w731]
          tunnel: w584 -> [_ w730]
          tunnel: w299 -> [_ w729]
          tunnel: w300 -> [_ w728]
          tunnel: [FALSE ("Polycold 1 Status") w730] -> w517
          tunnel: [w726 w735] -> w511
          tunnel: [w726 w734] -> w510
          tunnel: [w726 w733] -> w509
          tunnel: [w726 w732] -> w508
          frame False {
            w726 = 0.0 ("index")
          }
          frame True {
            n82 = shared-variable "MPR1\\Real-Time Library.lvlib\\Polycold 2 Status"() -> (w744:bool)  [unwired: 1 in, 1 out]
            n83 = Select(t=0.0 ("index"), s=w731, f=12.0 ("index")) -> (s? t:f=w733:dbl)
            n84 = Select(t=0.0 ("index"), s=w729, f=10.0 ("index")) -> (s? t:f=w735:dbl)
            n85 = Equal?(x=w744, y=w730) -> (x = y?=w745:bool)
            n86 = Select(t=0.0 ("index"), s=w728, f=11.0 ("index")) -> (s? t:f=w734:dbl)
            n87 = Select(t=0.0 ("index"), s=w745, f=13.0 ("index")) -> (s? t:f=w732:dbl)
          }
        }
        n88 = Array Subset(array=w372, length=4) -> (w499:bool[])  [unwired: 1 in]
        n89 = Equal?(x=u32 13, y=w414) -> (x = y?=w407:bool)
        n90 = Equal?(x=u32 13, y=w389) -> (x = y?=w396:bool)
        n91 = Equal?(x=w564, y=w555) -> (x = y?=w567:bool)
        n92 = Not Equal?(x=w555, y=w554) -> (x != y?=w568:bool)
        n93 = Not Equal?(x=w557, y=w556) -> (x != y?=w569:bool)
        n94 = Equal To 0?(x=w363) -> ()  [unwired: 1 out]
        n95 = VISA Read(VISA resource name=w423, byte count=w414, error in (no error)=w422) -> (VISA resource name out=w418:refnum<visa-resource-name>, read buffer=w411:string, error out=w419:errorcluster)  [unwired: 1 out]
        n96 = VISA Read(VISA resource name=w384, byte count=w389, error in (no error)=w385) -> (VISA resource name out=w379:refnum<visa-resource-name>, read buffer=w392:string, error out=w378:errorcluster)  [unwired: 1 out]
        n97 = Equal?(x=w556, y=w565) -> (x = y?=w570:bool)
        n98 = Array Subset(array=w427, length=10 ("index")) -> (w425:bool[])  [unwired: 1 in]
        n99 = VISA Read(VISA resource name=w365, byte count=w363, error in (no error)=w364) -> (VISA resource name out=w362:refnum<visa-resource-name>, read buffer=w360:string, error out=w361:errorcluster)  [unwired: 1 out]
        n100 = Not And(1:w568, 2:w567) -> (0:w566:bool)
        n101 = Not And(1:w570, 2:w569) -> (0:w571:bool)
        n102 = And(x="Heaters In Use?", y=w530) -> (x .and. y?=w527:bool)
        n103 = And(x="Ballast Bottle \nHeater in use?", y=w462) -> (x .and. y?=w464:bool)
        n104 = And(x="Xenon Heater\nIn Use?", y=w327) -> (x .and. y?=w325:bool)
        n105 = Replace Array Subset(array=w436, new element #1=w429, index #1=24 ("index"), new element #2=w425, index #2=34 ("index")) -> (w435:bool[])
        n106 = Select(t=2.0 ("index"), s=w527, f=0.0 ("index")) -> (s? t:f=w519:dbl)
        n107 = String Subset(string=w411, offset (0)=9, length (rest)=2 ("length (rest)")) -> (substring=w415:string)
        n108 = Select(t=20.0 ("index"), s=w566, f=0.0 ("index")) -> (s? t:f=w549:dbl)
        n109 = Select(t=42.0 ("index"), s=w464, f=0.0 ("index")) -> (s? t:f=w459:dbl)
        n110 = Select(t=63.0 ("index"), s=w325, f=0.0 ("index")) -> (s? t:f=w313:dbl)
        n111 = Select(t=19.0 ("index"), s=w571, f=0.0 ("index")) -> (s? t:f=w550:dbl)
        n112 = String Subset(string=w392, offset (0)=9, length (rest)=2 ("length (rest)")) -> (substring=w388:string)
        n113 = And(x="Heaters In Use?", y=w529) -> (x .and. y?=w526:bool)
        n114 = String Subset(string=w360, offset (0)=1, length (rest)=w354) -> (substring=w352:string)
        n115 = String Subset(string=w360, offset (0)=11, length (rest)=w354) -> (substring=w351:string)
        n116 = String Subset(string=w360, offset (0)=21, length (rest)=w354) -> (substring=w350:string)
        n117 = String Subset(string=w360, offset (0)=31, length (rest)=w354) -> (substring=w349:string)
        n118 = String Subset(string=w360, offset (0)=41, length (rest)=w354) -> (substring=w348:string)
        n119 = Greater?(x=w445, y=0.1) -> (0:w448:bool)
        n120 = Greater?(x=w335, y=0.1) -> (0:w333:bool)
        n121 = Equal?(x=w415, y="lb") -> (x = y?=w406:bool)
        n122 = Select(t=3.0 ("index"), s=w526, f=0.0 ("index")) -> (s? t:f=w520:dbl)
        n123 = Equal?(x=w388, y="lb") -> (x = y?=w397:bool)
        n124 = Select(t=0.0, s=w462, f=w445) -> (s? t:f=w460:dbl)
        n125 = Select(t=0.0, s=w327, f=w335) -> (s? t:f=w315:dbl)
        n126 = Select(t=0.0, s=w529, f=w536) -> (s? t:f=w537:dbl)
        n127 = Select(t=0.0, s=w530, f=w540) -> (s? t:f=w539:dbl)
        n128 = Replace Array Subset(array=w496, new element #1=w519, index #1=1 ("offset"), new element #2=w520, index #2=2 ("offset")) -> (w495:dbl[])
        n129 = Replace Array Subset(array=w495, new element #1=w515, index #1=5 ("index"), new element #2=w514, index #2=6 ("index"), new element #3=w513, index #3=7 ("index"), new element #4=w512, index #4=8 ("index"), new element #5=w511, index #5=9 ("index"), new element #6=w510, index #6=10 ("index"), new element #7=w509, index #7=11 ("index"), new element #8=w508, index #8=12 ("index"), new element #9=w507, index #9=13 ("index"), new element #10=w506, index #10=14 ("index"), new element #11=w505, index #11=15 ("index"), new element #12=w504, index #12=16 ("index")) -> (w494:dbl[])
        n130 = Replace Array Subset(array=w435, new element #1=w518, index #1=4 ("index"), new element #2=w517, index #2=5 ("index"), new element #3=w516, index #3=6 ("index"), new element #4=w371, index #4=7 ("index"), new element #5=w370, index #5=8 ("index"), new element #6=w305, index #6=9 ("index")) -> (w497:bool[])
        n131 = case shown="True" w448 {
          tunnel: w446 -> [w650 w657]
          tunnel: w445 -> [_ w656]
          tunnel: [w648 w651] -> w443
          frame False {
            n132 = Greater?(x=w650, y=0.5) -> (0:w648:bool)
          }
          frame True {
            n133 = Divide(x=w657, y=w656) -> (x/y=w655:dbl)
            n134 = In Range and Coerce(upper limit=3.5 ("lower limit"), x=w655, lower limit=3.0) -> (In Range?=w652:bool)  [unwired: 1 out]
            n135 = Not(x=w652) -> (.not. x?=w651:bool)
          }
        }
        n136 = case shown="True" w333 {
          tunnel: w316 -> [w605 w612]
          tunnel: w335 -> [_ w611]
          tunnel: [w603 w606] -> w336
          frame False {
            n137 = Greater?(x=w605, y=0.5) -> (0:w603:bool)
          }
          frame True {
            n138 = Divide(x=w612, y=w611) -> (x/y=w610:dbl)
            n139 = In Range and Coerce(upper limit=50.0 ("lower limit"), x=w610, lower limit=0.001) -> (In Range?=w607:bool)  [unwired: 1 out]
            n140 = Not(x=w607) -> (.not. x?=w606:bool)
          }
        }
        n141 = And(x=w406, y=w407) -> (x .and. y?=w403:bool)
        n142 = And(x=w397, y=w396) -> (x .and. y?=w400:bool)
        n143 = Subtract(x=w455, y=w446) -> (x-y=w454:dbl)
        n144 = Subtract(x=w308, y=w316) -> (x-y=w328:dbl)
        n145 = String Subset(string=w411, length (rest)=8 ("length (rest)")) -> (substring=w410:string)  [unwired: 1 in]
        n146 = String Subset(string=w392, length (rest)=8 ("length (rest)")) -> (substring=w393:string)  [unwired: 1 in]
        n147 = Replace Array Subset(array=w353, new element #1=w352, new element #2=w351, new element #3=w350, index #3=2 ("index"), new element #4=w349, index #4=3 ("index"), new element #5=w348, index #5=4 ("index")) -> (w344:string[])  [unwired: 2 in]
        n148 = Absolute Value(x=w454) -> (abs(x)=w453:dbl)
        n149 = Absolute Value(x=w328) -> (abs(x)=w329:dbl)
        n150 = Select(t=1.0, s="Xenon Heater\nIn Use?", f=0.0 ("t")) -> (s? t:f=w307:dbl)
        n151 = Greater?(x=w453, y=10.0) -> (0:w449:bool)
        n152 = Greater?(x=w329, y=0.3) -> (0:w332:bool)
        n153 = Select(t=0.0 ("index"), s=w403, f=0.0 ("index")) -> (s? t:f=w402:dbl)
        n154 = Select(t=0.0 ("index"), s=w400, f=0.0 ("index")) -> (s? t:f=w380:dbl)
        n155 = Fract/Exp String To Number(string=w410, default (0 dbl)=-1.2 ("default (0 DBL)")) -> (number=w401:dbl)  [unwired: 2 in, 1 out]
        n156 = Fract/Exp String To Number(string=w344) -> (number=w343:dbl[])  [unwired: 3 in, 1 out]
        n157 = And(x="Ballast Bottle \nHeater in use?", y=w449) -> (x .and. y?=w450:bool)
        n158 = And(x="Xenon Heater\nIn Use?", y=w332) -> (x .and. y?=w331:bool)
        n159 = And(x=w443, y="Ballast Bottle \nHeater in use?") -> (x .and. y?=w439:bool)
        n160 = And(x=w336, y="Xenon Heater\nIn Use?") -> (x .and. y?=w340:bool)
        n161 = Fract/Exp String To Number(string=w393, default (0 dbl)=-1.2 ("default (0 DBL)")) -> (number=w381:dbl)  [unwired: 2 in, 1 out]
        n162 = Select(t=44.0 ("index"), s=w450, f=0.0 ("index")) -> (s? t:f=w438:dbl)
        n163 = Select(t=64.0 ("index"), s=w331, f=0.0 ("index")) -> (s? t:f=w312:dbl)
        n164 = Select(t=45.0 ("index"), s=w439, f=0.0 ("index")) -> (s? t:f=w437:dbl)
        n165 = Select(t=65.0 ("index"), s=w340, f=0.0 ("index")) -> (s? t:f=w311:dbl)
      }
      frame #1 {
        w834 = 5 ("offset (0)")
        w898 = 0.03027 ("y")
        w1044 = refnum<k21> "FieldPoint\\MPR1\\Digital Voltage Output Module 1\\Pump Stop c15"  # FieldPoint IO Point
        w1079 = 5 ("offset (0)")
        w1657 = -1 ("Manometer\nOn/Off\n Threshold")
        w1147 = 10.0 ("y")
        w1213 = refnum<k21> "FieldPoint\\MPR1\\Analog Voltage Input Module 2\\All"  # FieldPoint IO Point
        w1214 = refnum<k21> "FieldPoint\\MPR1\\Digital Voltage Output Module 1\\Pumpout Cart Valve 2 c2"  # FieldPoint IO Point
        w1215 = refnum<k21> "FieldPoint\\MPR1\\Digital Voltage Output Module 1\\Pumpout Cart Valve 1 c0"  # FieldPoint IO Point
        w1234 = refnum<k21> "FieldPoint\\MPR1\\Digital Voltage Output Module 1\\Vent to At Valve c12"  # FieldPoint IO Point
        w1235 = refnum<k21> "FieldPoint\\MPR1\\Digital Voltage Output Module 1\\Relief to Wess Valves c13"  # FieldPoint IO Point
        w1237 = refnum<k21> "FieldPoint\\MPR1\\Digital Voltage Output Module 1\\Cryost Vapor Fill Valve c14"  # FieldPoint IO Point
        w1240 = refnum<k21> "FieldPoint\\MET1\\cFP-TC-120 @2\\All"  # FieldPoint IO Point
        w1247 = refnum<k21> "FieldPoint\\MET1\\cFP-TC-120 @1\\All"  # FieldPoint IO Point
        w1271 = refnum<k21> "FieldPoint\\MET1\\cFP-TC-120 @7\\All"  # FieldPoint IO Point
        w1272 = refnum<k21> "FieldPoint\\MET1\\cFP-TC-120 @6\\All"  # FieldPoint IO Point
        w1287 = refnum<k21> "FieldPoint\\MPR1\\Thermocouple Module 2 (Slot 2)\\All"  # FieldPoint IO Point
        w1288 = refnum<k21> "FieldPoint\\MPR1\\Thermocouple Module 1 (Slot 1)\\All"  # FieldPoint IO Point
        w1312 = refnum<k21> "FieldPoint\\MPR1\\Thermocouple Module 3 (Slot 3)\\All"  # FieldPoint IO Point
        w1321 = refnum<k21> "FieldPoint\\MPR1\\Analog Current Input Module 1\\All"  # FieldPoint IO Point
        w1329 = refnum<k21> "FieldPoint\\MPR1\\Analog Voltage Input Module 1\\All"  # FieldPoint IO Point
        w1331 = refnum<k21> "FieldPoint\\MET1\\cFP-TC-120 @5\\All"  # FieldPoint IO Point
        w860 = 4 ("length")
        w1389 = 5 ("offset (0)")
        w1438 = 5 ("offset (0)")
        (unwired) 4 ("element")
        w1668 = "IOUT?\r\n" ("string to write")
        w1244 = 4 ("length")
        w1663 = FALSE
        w1805 = 0.0 ("y")
        # "Recirculation Pump"
        # "Xenon Heater"
        # "Turn off heater when overpressure???"
        # "Heater for Condenser Control"
        # "Inclinemeter Conversion"
        # "Logic for HFE Valves"
        # "Pumpout Cart Valve 2 Signal"
        # "Pumpout Cart Valve 1 Signal"
        # "GRAB TC Information for Polycold 1"
        # "GRAB TC Information for Cryostat"
        # "CRYOSTAT HEATERS CONTROLS"
        # "Turbopump #2 Status"
        # "Turbopump #1 Status"
        # "PT503"
        # "PT102"
        # "PT101"
        # "TC Gauge Valve 2"
        # "TC Gauge Valve 1"
        # "From CC Gauge\n(pumpout cart)"
        # "Polycold 3 Signals"
        # "Polycold 2 Signals"
        # "Polycold 1 Signals"
        # "Pumpout Cart"
        # "Send the Values to the Monitoring PC"
        # "Grabbing the Dust Counter Values"
        # "Heater for HFE Ballast Bottle"
        # "Feed and Bleed Control"
        # "Fridges for Inner Cryostat Control"
        n166 = property class="Instr"(reference=w1752, error in=w1751) -> (reference out=w1753:refnum<visa-resource-name>, error out=w1754:errorcluster, "Serial Settings:Number of Bytes at Serial Port"=w1747:u32)
        n167 = call <vilib>:"FP Read (Float Array -IO).vi"("FieldPoint IO Point In"=w1272) -> ("values"=w1270:dbl[])  [unwired: 11 in, 3 out]
        n168 = call <vilib>:"FP Read (Float Array -IO).vi"("FieldPoint IO Point In"=w1271) -> ("values"=w1269:dbl[])  [unwired: 11 in, 3 out]
        n169 = shared-variable "MPR2\\MPR2 Library.lvlib\\Data MPR 2"() -> (w1224:dbl[])  [unwired: 1 in, 1 out]
        n170 = call "TempConvert.vi"("All type T\nTC data \nfrom module"=w1270) -> ("Temperature (K)"=w855:dbl[])
        n171 = call "TempConvert.vi"("All type T\nTC data \nfrom module"=w1269) -> ("Temperature (K)"=w931:dbl[])
        n172 = VISA Write(VISA resource name=w1145, write buffer="#000F\r", error in (no error)=w1144) -> (VISA resource name out=w1143:refnum<visa-resource-name>, error out=w1142:errorcluster)  [unwired: 1 out]
        n173 = call <vilib>:"FP Read (Float Array -IO).vi"("FieldPoint IO Point In"=w1288) -> ("values"=w1285:dbl[])  [unwired: 11 in, 3 out]
        n174 = call "TempConvert.vi"("All type T\nTC data \nfrom module"=w1285) -> ("Temperature (K)"=w1422:dbl[])
        n175 = Array Subset(array=w931, length=5) -> (w1263:dbl[])  [unwired: 1 in]
        n176 = call <vilib>:"FP Read (Float Array -IO).vi"("FieldPoint IO Point In"=w1329) -> ("values"=w1185:dbl[])  [unwired: 11 in, 3 out]
        n177 = Index Array(array=w855, index=7) -> (element=w1264:dbl)
        n178 = call <vilib>:"FP Read (Float Array -IO).vi"("FieldPoint IO Point In"=w1287) -> ("values"=w1286:dbl[])  [unwired: 11 in, 3 out]
        n179 = Array Subset(array=w1224, length=4) -> (w1275:dbl[])  [unwired: 1 in]
        n180 = Array Subset(array=w1224, index=11, length=4) -> (w1278:dbl[])
        n181 = Array Subset(array=w1224, index=17, length=4) -> (w767:dbl[])
        n182 = Array Subset(array=w1224, index=5, length=6) -> (w1229:dbl[])
        n183 = Array Subset(array=w855, length=7) -> (w1226:dbl[])  [unwired: 1 in]
        n184 = call "TempConvert.vi"("All type T\nTC data \nfrom module"=w1286) -> ("Temperature (K)"=w1615:dbl[])
        n185 = Array Subset(array=w1185, length=2) -> (w1298:dbl[])  [unwired: 1 in]
        n186 = Index Array(array=w1185, index=12) -> (element=w1297:dbl)
        n187 = Index Array(array=w1185, index=13) -> (element=w1294:dbl)
        n188 = Array Subset(array=w1185, index=5, length=6) -> (w1291:dbl[])
        n189 = Index Array(array=w1185, index=11) -> (element=w1184:dbl)
        n190 = Index Array(array=w767) -> (element=w766:dbl)  [unwired: 1 in]
        n191 = Index Array(array=w1224, index #1=15 ("index"), index #2=16 ("length")) -> (element #1=w1216:dbl, element #2=w1217:dbl)
        n192 = expression code="4.0928*(x-2.5)+0.0132*((x-2.5)**2)+0.0146*((x-2.5)**3)-0.0028*((x-2.5)**4)-0.0022*((x-2.5)**5)"(w1294) -> (w1295:dbl)
        n193 = Index Array(array=w1275, index=3) -> (element=→"Actual":dbl)
        n194 = Index Array(array=w1224, index=4) -> (element=w1248:dbl)
        n195 = expression code="x*500"(w1297) -> (w1296:dbl)
        n196 = call <vilib>:"FP Read (Float Array -IO).vi"("FieldPoint IO Point In"=w1312) -> ("values"=w1232:dbl[])  [unwired: 11 in, 3 out]
        n197 = Index Array(array=w855, index=5) -> (element=w854:dbl)
        n198 = expression code="x*500"(w1184) -> (w1179:dbl)
        n199 = expression code="x*500"(w1291) -> (w1182:dbl[])
        n200 = expression code="x*500"(w1298) -> (w1340:dbl[])
        n201 = Equal?(x="dP Offset 2 (torr)", y="dP Offset 1 (torr)") -> (x = y?=w804:bool)
        n202 = call <vilib>:"FP Read (Float Array -IO).vi"("FieldPoint IO Point In"=w1213) -> ("values"=w1212:dbl[])  [unwired: 11 in, 3 out]
        n203 = Index Array(array=w1182, index=2) -> (element=w1178:dbl)
        n204 = Select(t=FALSE, s="Yoyo method while in\nAutomatic?", f=w804) -> (s? t:f=w803:bool)
        n205 = call-poly <vilib>:"FP Read (Polymorphic).vi"("FieldPoint IO Point In"=w1331) -> ("values"=w850:dbl[])  [unwired: 11 in, 3 out]
        n206 = call <vilib>:"FP Read (Float Array -IO).vi"("FieldPoint IO Point In"=w1247) -> ("values"=w1246:dbl[])  [unwired: 11 in, 3 out]
        n207 = call <vilib>:"FP Read (Float Array -IO).vi"("FieldPoint IO Point In"=w1240) -> ("values"=w1239:dbl[])  [unwired: 11 in, 3 out]
        n208 = Select(t="dP Offset 2 (torr)", s=w803, f=w823) -> (s? t:f=w793:dbl)
        "Actual dP Offset (torr)" <- w793
        n209 = Index Array(array=w850) -> (element=w849:dbl)  [unwired: 1 in]
        n210 = Select(t=21.0 ("index"), s=w1682, f=0.0 ("index")) -> (s? t:f=w923:dbl)
        n211 = Greater Or Equal?(x="Heater Output \nHigh Limit (Volts)", y="Heater Output \nLow Limit (Volts)") -> (x >= y?=w1677:bool)
        n212 = VISA Read(VISA resource name=w1753, byte count=w1747, error in (no error)=w1754) -> (VISA resource name out=w1749:refnum<visa-resource-name>, read buffer=w1724:string, error out=w1748:errorcluster)  [unwired: 1 out]
        n213 = Negate(x="High dP limit for Yoyo") -> (-x=w799:dbl)
        n214 = Split 1D Array(array=w1226, index=4) -> (first subarray=w1225:dbl[], second subarray=w1218:dbl[])
        n215 = Equal?(x=w1747, y=u32 50) -> (x = y?=w1729:bool)
        n216 = Select(t=18.0 ("index"), s=w1316, f=0.0 ("index")) -> (s? t:f=w1597:dbl)
        n217 = Negate(x="Low dP limit for Yoyo") -> (-x=w800:dbl)
        n218 = call "TempConvert.vi"("All type T\nTC data \nfrom module"=w850) -> ("Temperature (K)"=w861:dbl[])
        n219 = Select(t="Heater Output \nHigh Limit (Volts)", s=w1677, f="Heater Output \nLow Limit (Volts)") -> (s? t:f=w1676:dbl)
        n220 = Greater Or Equal?(x="High", y="Low") -> (x >= y?=w1759:bool)
        n221 = Select(t=1.0 ("index"), s="Condenser \nin Use?", f=0.0 ("index")) -> (s? t:f=w943:dbl)
        n222 = Select(t=1.0 ("index"), s="Reinitialize\nCondenser PID", f=0.0 ("index")) -> (s? t:f=w942:dbl)
        n223 = Replace Array Subset(array=w1289, new element #1=w943, new element #2=w942, index #2=1 ("index")) -> (w940:dbl[])  [unwired: 1 in]
        n224 = Array Subset(array=w861, length=w860) -> (w900:dbl[])  [unwired: 1 in]
        n225 = call <vilib>:"FP Read (Float Array -IO).vi"("FieldPoint IO Point In"=w1321, "Type"=dbl[] []) -> ("values"=w890:dbl[])  [unwired: 10 in, 3 out]
        n226 = In Range and Coerce(upper limit=10 ("element"), x=w771, lower limit=1) -> (In Range?=w772:bool)  [unwired: 1 out]
        n227 = Negate(x="delta (Dead band)\n(torr)") -> (-x=w1808:dbl)
        n228 = String Subset(string=w1724, offset (0)=0, length (rest)=1 ("length (rest)")) -> (substring=w1731:string)
        n229 = Select(t="High", s=w1759, f="Low") -> (s? t:f=w1758:dbl)
        n230 = property on="Heater Output \nHigh Limit (Volts)" class="DigNum (strict)"("Value"=w1676) -> ()  [unwired: 2 in, 2 out]
        n231 = shared-variable "MPR1\\Real-Time Library.lvlib\\Boolean Data for MR2"(w940) -> ()  [unwired: 1 in, 1 out]
        n232 = Bundle("Heater Output \nLow Limit (Volts)"=w1676, "Heater Output \nLow Limit (Volts)"="Heater Output \nLow Limit (Volts)") -> (w1675:T6)  [unwired: 1 in]
        n233 = Equal To 0?(x="Ring") -> (x = 0?=w1107:bool)
        n234 = Equal?(x="Ring", y=u16 1) -> (x = y?=w1138:bool)
        n235 = Equal?(x="Ring", y=u16 2) -> (x = y?=w1103:bool)
        n236 = Index Array(array=w861, index=w860) -> (element=w859:dbl)
        n237 = call "TempConvert.vi"("All type T\nTC data \nfrom module"=w1239) -> ("Temperature (K)"=w1238:dbl[])
        n238 = call "TempConvert.vi"("All type T\nTC data \nfrom module"=w1246) -> ("Temperature (K)"=w1245:dbl[])
        n239 = call "TempConvert.vi"("All type T\nTC data \nfrom module"=w1232) -> ("Temperature (K)"=w1566:dbl[])
        n240 = Equal?(x="=", y=w1731) -> (x = y?=w1728:bool)
        n241 = property on="High" class="DigNum (strict)"("Value"=w1758) -> ()  [unwired: 2 in, 2 out]
        n242 = Index Array(array=w890, index=10) -> (element=w891:dbl)
        n243 = String Subset(string=w1724, offset (0)=10, length (rest)=5 ("length (rest)")) -> (substring=w1435:string)
        n244 = And(x=w1729, y=w1728) -> (x .and. y?=w1732:bool)
        n245 = String Subset(string=w1724, offset (0)=4, length (rest)=5 ("length (rest)")) -> (substring=w1436:string)
        n246 = Array Subset(array=w1245, length=w1244) -> (w1547:dbl[])  [unwired: 1 in]
        n247 = Array Subset(array=w1245, index=w1244, length=w1244) -> (w1242:dbl[])
        n248 = expression code="497/.016*x-497/4"(w891) -> (w889:dbl)
        n249 = Select(t=1.0, s="Enter Liquid\nLevel Manually?", f=0.0) -> (s? t:f=w879:dbl)
        n250 = Index Array(array=w931, index #1=5 ("index"), index #2=6 ("index")) -> (element #1=w1311:dbl, element #2=w1354:dbl)
        n251 = String Subset(string=w1724, offset (0)=22, length (rest)=5 ("length (rest)")) -> (substring=w1433:string)
        n252 = String Subset(string=w1724, offset (0)=16, length (rest)=5 ("length (rest)")) -> (substring=w1434:string)
        n253 = Index Array(array=w1340, index #1=1 ("index"), index #2=0 ("index")) -> (element #1=w1338:dbl, element #2=w1337:dbl)
        n254 = Unbundle("Cryostat Heater PID Gains") -> ("Proportional gain (Kc)"=w1608:dbl, "Integral time (Ti, min)"=w1607:dbl, "Derivative time (Td, min)"=w1606:dbl)
        n255 = Subtract(x=w1179, y=w1178) -> (x-y=w1823:dbl)
        n256 = Index Array(array=w1212, index #1=12 ("index"), index #2=13 ("index"), index #3=4 ("index"), index #4=7 ("index"), index #5=0 ("index"), index #6=9 ("index"), index #7=1 ("index"), index #8=14 ("index"), index #9=15 ("index")) -> (element #1=w907:dbl, element #2=w906:dbl, element #3=w1170:dbl, element #4=w1684:dbl, element #5=w1575:dbl, element #6=w1683:dbl, element #7=w1573:dbl, element #8=w908:dbl, element #9=w909:dbl)
        n257 = Multiply(x=w907, y=500.0) -> (x*y=w919:dbl)
        n258 = Multiply(x=w906, y=500.0) -> (x*y=w917:dbl)
        n259 = Divide(x=w919, y=w898) -> (x/y=w918:dbl)
        n260 = Divide(x=w917, y=w898) -> (x/y=w915:dbl)
        n261 = Multiply(x=w909, y=250.0) -> (x*y=w911:dbl)
        n262 = Multiply(x=w908, y=500.0) -> (x*y=w913:dbl)
        n263 = Divide(x=w911, y=w898) -> (x/y=w794:dbl)
        n264 = Divide(x=w913, y=w898) -> (x/y=w912:dbl)
        n265 = Compound Arithmetic op=ADD(w918, w915, w912, w794) -> ()  [unwired: 1 out]
        n266 = Subtract(x=w1338, y=w1337) -> (x-y=w1822:dbl)
        n267 = Subtract(x="PT #(After Purifier)", y="PT #(Before Purifier)") -> (x-y=w1024:i32)
        n268 = Select(t=1.0, s="HFE head disable", f=0.0) -> (s? t:f=w874:dbl)
        n269 = Index Array(array=w1185, index #1=2 ("index"), index #2=3 ("index"), index #3=4 ("index")) -> (element #1=w1314:dbl, element #2=w1313:dbl, element #3=w1315:dbl)
        n270 = case shown="False" "HFE head disable" {
          tunnel: TRUE ("x > y?") -> [w1831 _]
          tunnel: [w1831 FALSE] -> w885
          frame False {
          }
          frame True {
          }
        }
        n271 = Index Array(array=w890, index=2) -> (element=w1173:dbl)
        n272 = Array Subset(array=w890, length=2) -> (w1172:dbl[])  [unwired: 1 in]
        n273 = Index Array(array=w890, index=9) -> (element=w1344:dbl)
        n274 = Array Subset(array=w890, index=6, length=2) -> (w1407:dbl[])
        n275 = Index Array(array=w890, index=5) -> (element=w1400:dbl)
        n276 = Index Array(array=w890, index=8) -> (element=w1408:dbl)
        n277 = Array Subset(array=w890, index=3, length=2) -> (w1406:dbl[])
        n278 = Absolute Value(x=w1822) -> (abs(x)=w1339:dbl)
        n279 = Absolute Value(x=w1823) -> (abs(x)=w1180:dbl)
        n280 = String Subset(string=w1724, offset (0)=28, length (rest)=5 ("length (rest)")) -> (substring=w1432:string)
        n281 = String Subset(string=w1724, offset (0)=34, length (rest)=5 ("length (rest)")) -> (substring=w1431:string)
        n282 = expression code="(x-0.004)*40373"(w1172) -> (w1086:dbl[])
        n283 = expression code="88.851*1000*x-1008.6"(w1173) -> (w1087:dbl)
        n284 = In Range and Coerce(upper limit="High Limit\nfor dP Gauge", x=w1087, lower limit="Low Limit\nfor dP Gauge") -> (In Range?=w1809:bool)  [unwired: 1 out]
        n285 = Select(t=0.0 ("index"), s=w1809, f=31.0 ("index")) -> (s? t:f=w1628:dbl)
        n286 = shared-variable "MPR2\\MPR2 Library.lvlib\\Alarm MPR 2"() -> (w953:dbl[])  [unwired: 1 in, 1 out]
        n287 = Divide(x=w1684, y=2.0) -> (x/y=w1576:dbl)
        n288 = Divide(x=w1683, y=2.0) -> (x/y=w1574:dbl)
        n289 = Not(x=w1603) -> (.not. x?=w1660:bool)
        n290 = Greater?(x=w1339, y="2 HFE \nManometers \nMax Var (torr)") -> (0:w1814:bool)
        n291 = expression code="50/.016*x-50/4"(w1406) -> (w1405:dbl[])
        n292 = expression code="50/.016*x-50/4"(w1407) -> (w905:dbl[])
        n293 = expression code="497/.016*x-497/4"(w1344) -> (w870:dbl)
        n294 = Add(x=w870, y=738.5) -> (x+y=w868:dbl)
        n295 = expression code="50/.016*x-50/4"(w1408) -> (w812:dbl)
        n296 = Greater?(x=w1180, y="2 Xe Manometers \nMax Var (torr)") -> (0:w1813:bool)
        n297 = Absolute Value(x=w1024) -> (abs(x)=w1023:i32)
        n298 = Multiply(x=w1575, y=w1147) -> (x*y=w1149:dbl)
        n299 = expression code="(x-0.2)/5*3000"(w1170) -> (w1169:dbl)
        n300 = Replace Array Subset(array=w1423, new element #1=w1436, index #1=0 ("length (rest)"), new element #2=w1435, index #2=1 ("length (rest)"), new element #3=w1434, index #3=2 ("length (rest)"), new element #4=w1433, index #4=3 ("length (rest)"), new element #5=w1432, index #5=4 ("length (rest)"), new element #6=w1431, index #6=5 ("length (rest)")) -> (w1424:string[])
        n301 = Quotient & Remainder(x=w1315, y=1 ("offset (0)")) -> (x-y*floor(x/y)=w1719:dbl, floor(x/y)=w1718:dbl)
        n302 = Index Array(array=w905, index #2=1 ("index")) -> (element #1=w901:dbl, element #2=w811:dbl)  [unwired: 1 in]
        n303 = Multiply(x=w901, y=51.71) -> (x*y=w903:dbl)
        n304 = Quotient & Remainder(x=w1313, y=1 ("offset (0)")) -> (x-y*floor(x/y)=w1709:dbl, floor(x/y)=w1708:dbl)
        n305 = Quotient & Remainder(x=w1314, y=1 ("offset (0)")) -> (x-y*floor(x/y)=w1714:dbl, floor(x/y)=w1713:dbl)
        n306 = case shown="False" w1813 {
          tunnel: w1179 -> [_ w2089]
          tunnel: [w2085 w2087] -> w1146
          tunnel: w1178 -> [w2085 w2088]
          tunnel: [0.0 ("index") 37.0 ("index")] -> w1627
          frame False {
          }
          frame True {
            n307 = Max & Min(x=w2089, y=w2088) -> (max(x,y)=w2087:dbl)  [unwired: 1 out]
          }
        }
        n308 = Negate(x="|dP| Maximum\n(torr)") -> (-x=w1131:dbl)
        n309 = case shown="True" w1814 {
          tunnel: [w2079 w2083] -> w865
          tunnel: [0.0 ("index") 38.0 ("index")] -> w1626
          tunnel: w1338 -> [_ w2082]
          tunnel: w1337 -> [w2079 w2081]
          frame False {
          }
          frame True {
            n310 = Max & Min(x=w2082, y=w2081) -> (max(x,y)=w2083:dbl)  [unwired: 1 out]
          }
        }
        "Actual" <- w865
        n311 = Greater?(x=w865, y="HFE Relief to\nAtmosphere\nThreshold (torr)") -> (0:w1112:bool)
        n312 = Greater?(x=w865, y="HFE Relief to\nWessington \nThreshold (torr)") -> (0:w1307:bool)
        n313 = Less?(x=w865, y="HFE Vapor Fill\nSet Point (torr)") -> (x < y?=w1310:bool)
        n314 = Select(t=w1310, s=w1138, f=FALSE) -> (s? t:f=w1135:bool)
        n315 = Greater?(x=w865, y=w903) -> (0:w904:bool)
        n316 = Or(x=w1135, y=w1103) -> (x .or. y?=w1136:bool)
        n317 = Multiply(x=w865, y=0.9717) -> (x*y=w867:dbl)
        n318 = Subtract(x=w868, y=w867) -> (x-y=w864:dbl)
        n319 = Select(t="Manual Liquid\nLevel (cm)", s="Enter Liquid\nLevel Manually?", f=w864) -> (s? t:f=w871:dbl)
        n320 = expression code="x*517.14/497/0.0075"(w871) -> (w895:dbl)
        n321 = Greater?(x=w871, y=63.5) -> ()  [unwired: 1 out]
        n322 = Multiply(x=w1147, y=w1573) -> (x*y=w1148:dbl)
        n323 = Subtract(x=w812, y=w811) -> (x-y=w810:dbl)
        n324 = Hexadecimal String To Number(string=w1424) -> (number=w1727:u32[])  [unwired: 2 in, 1 out]
        n325 = expression code="(x+0.1)/.11"(w1719) -> (w1717:dbl)
        n326 = expression code="10**(x-11)"(w1718) -> (w1716:dbl)
        n327 = Greater Or Equal?(x="Xenon Heater \nOutput \nHigh Limit", y="Xenon Heater \nOutput \nLow Limit") -> (x >= y?=w1020:bool)
        n328 = call-poly <vilib>:"PID.vi"("reinitialize? (F)"="Reinitialize\nHeater PID", "output range"=w1675, "PID gains"="Cryostat Heater PID Gains", "process variable"=w1216, "setpoint"="Temperature\nSet Point (K)") -> ("output"=w1666:dbl)  [unwired: 5 in, 1 out]
        n329 = expression code="(x+0.1)/.11"(w1709) -> (w1707:dbl)
        n330 = expression code="10**(x-4)"(w1708) -> (w1706:dbl)
        n331 = Array Subset(array=w953, index=2, length=3) -> (w951:dbl[])
        n332 = expression code="(x+0.1)/.11"(w1714) -> (w1712:dbl)
        n333 = expression code="10**(x-4)"(w1713) -> (w1711:dbl)
        n334 = Greater Or Equal?(x="Recirc. Pump \nOutput \nHigh Limit", y="Recirc. Pump \nOutput \nLow Limit") -> (x >= y?=w1026:bool)
        n335 = Greater?(x=w1023, y="Max |dP|\nacross purifier") -> (0:w1022:bool)
        n336 = Less?(x="Heater Temperature\nHigh Cutoff Limit (K)", y=w1216) -> (x < y?=w1665:bool)
        n337 = Index Array(array=w905, index=1 ("element")) -> (element=w936:dbl)
        "Actual Pressure\n(psi)" <- w936
        n338 = expression code="-2.86*x + 2257"(w854) -> (w894:dbl)
        n339 = case shown="False" "Bleed 50?" {
          tunnel: [refnum<k21> "FieldPoint\\MPR1\\Digital Voltage Output Module 1\\V-X51 c8" ("FieldPoint IO Point") refnum<k21> "FieldPoint\\MPR1\\Digital Voltage Output Module 1\\V-X50 c7" ("FieldPoint IO Point")] -> w843
          tunnel: [refnum<k21> "FieldPoint\\MPR1\\Digital Voltage Output Module 1\\V-X50 c7" ("FieldPoint IO Point") refnum<k21> "FieldPoint\\MPR1\\Digital Voltage Output Module 1\\V-X51 c8" ("FieldPoint IO Point")] -> w842
          frame False {
          }
          frame True {
          }
        }
        n340 = Select(t="Xenon Heater \nOutput \nHigh Limit", s=w1020, f="Xenon Heater \nOutput \nLow Limit") -> (s? t:f=w1021:dbl)
        n341 = Multiply(x=100 ("index"), y=w1727) -> (x*y=w1726:u32[])
        n342 = Select(t="Recirc. Pump \nOutput \nHigh Limit", s=w1026, f="Recirc. Pump \nOutput \nLow Limit") -> (s? t:f=w1025:dbl)
        n343 = Replace Array Subset(array=w1569, new element #1="Heater Temperature\nHigh Cutoff Limit (K)", index #1=i16 53 ("precision (6)"), new element #2="Temperature\nSet Point (K)", index #2=i16 54 ("precision (6)"), new element #3=w1608, index #3=i16 55 ("precision (6)"), new element #4=w1607, index #4=i16 56 ("precision (6)"), new element #5=w1606, index #5=i16 57 ("precision (6)"), new element #6="Heater Output \nHigh Limit (Volts)", index #6=i16 58 ("precision (6)"), new element #7="Heater Output \nLow Limit (Volts)", index #7=i16 59 ("precision (6)")) -> (w1568:dbl[])
        n344 = Array Subset(array=w953, length=2) -> (w955:dbl[])  [unwired: 1 in]
        n345 = Multiply(x=w1717, y=w1716) -> (x*y=w922:dbl)
        n346 = Multiply(x=w1707, y=w1706) -> (x*y=w1571:dbl)
        n347 = Replace Array Subset(array=w1559, new element #1="Reinitialize\nHeater PID", index #1=i16 10 ("precision (6)"), new element #2=w1603, index #2=i16 11 ("precision (6)")) -> (w1199:bool[])
        n348 = Multiply(x=9.8 ("y"), y=0.635) -> (x*y=w887:dbl)
        n349 = property on="Xenon Heater \nOutput \nHigh Limit" class="DigNum (strict)"("Value"=w1021) -> ()  [unwired: 2 in, 2 out]
        n350 = Multiply(x=w1712, y=w1711) -> (x*y=w1572:dbl)
        n351 = property on="Recirc. Pump \nOutput \nHigh Limit" class="DigNum (strict)"("Value"=w1025) -> ()  [unwired: 2 in, 2 out]
        n352 = expression code="x*51.7/.97"(w810) -> (w809:dbl)
        n353 = Subtract(x=w809, y=w1111) -> (x-y=w1099:dbl)
        n354 = Less?(x=w809, y="Ballast Bottle Low\nLevel Alarm (cm)") -> (x < y?=w1056:bool)
        n355 = Multiply(x=w894, y=w887) -> (x*y=w893:dbl)
        n356 = Or(x=w1665, y=w1660) -> (x .or. y?=w1664:bool)
        n357 = Bundle("Xenon Heater \nOutput \nLow Limit"=w1021, "Xenon Heater \nOutput \nLow Limit"="Xenon Heater \nOutput \nLow Limit") -> (w1019:T7)  [unwired: 1 in]
        n358 = Select(t=56.0 ("index"), s="Manual Operation of HFE Valves?", f=0.0 ("index")) -> (s? t:f=w1120:dbl)
        n359 = case shown="True" w1732 {
          tunnel: w1726 -> [_ _]
          frame False {
          }
          frame True {
          }
        }
        n360 = Greater?(x=w922, y="CC Soft Threshold\nAlarm (Torr)") -> (0:w1705:bool)
        n361 = Bundle("Recirc. Pump \nOutput \nLow Limit"=w1025, "Recirc. Pump \nOutput \nLow Limit"="Recirc. Pump \nOutput \nLow Limit") -> (w1027:T8)  [unwired: 1 in]
        n362 = Greater?(x=w1572, y="TC 1/2 Soft Threshold\nAlarm (Torr)") -> (0:w1703:bool)
        n363 = Less?(x="Ballast Bottle\nOverpressure (psi)", y=w936) -> (x < y?=w1378:bool)
        n364 = Less?(x=w1146, y=w1657) -> (x < y?=w1723:bool)
        n365 = Less?(x=w865, y=w1657) -> (x < y?=w1722:bool)
        n366 = call-poly <vilib>:"PID.vi"("reinitialize? (F)"="Reinitialize\nRecirc. Pump PID", "output range"=w1027, "dt (s)"=w1372, "PID gains"="Recirc. Pump PID Gains", "process variable"=w1024, "setpoint"="dP across purifier\nset point value") -> ("output"=→"Recirc. Pump output":dbl)  [unwired: 4 in, 1 out]
        n367 = Select(t=0.0, s=w1664, f=w1666) -> (s? t:f=w828:dbl)
        n368 = Greater?(x=w1571, y="TC 1/2 Soft Threshold\nAlarm (Torr)") -> (0:w1704:bool)
        n369 = Or(x=w1723, y=w1722) -> (x .or. y?=w1721:bool)
        n370 = Compound Arithmetic op=OR(w1721, w1813, w1814) -> (w1810:bool)
        n371 = And(x=w1810, y=w1809) -> (x .and. y?=w1811:bool)
        n372 = Less?(x=w864, y="Cryostat Low Liquid\nLevel Alarm (cm)") -> (x < y?=w1050:bool)
        n373 = Greater Or Equal?(x="High", y="Low") -> (x >= y?=w1032:bool)
        n374 = Select(t=25.0 ("index"), s=w1703, f=0.0 ("index")) -> (s? t:f=w1578:dbl)
        n375 = Subtract(x=w1146, y=w865) -> (x-y=w872:dbl)
        n376 = Subtract(x=w872, y=w1087) -> (x-y=w1817:dbl)
        n377 = Absolute Value(x=w1817) -> (abs(x)=w1816:dbl)
        n378 = Greater?(x=w1816, y="Max diff between \ndP from gauge and\ndP from man. (torr)") -> (0:w1815:bool)
        n379 = Select(t=29.0 ("index"), s=w1815, f=0.0 ("index")) -> (s? t:f=w1630:dbl)
        n380 = Select(t=w1087, s=w1811, f=w872) -> (s? t:f=w896:dbl)
        n381 = case shown="True" w885 {
          tunnel: w896 -> [w1833 w1839]
          tunnel: [w1833 w1835] -> w807
          tunnel: w895 -> [_ w1840]
          tunnel: w893 -> [_ w1834]
          frame False {
          }
          frame True {
            n382 = expression code="x/0.0075"(w1839) -> (w1836:dbl)
            n383 = Subtract(x=w1836, y=w1840) -> (x-y=w1838:dbl)
            n384 = Add(x=w1834, y=w1838) -> (x+y=w1837:dbl)
            n385 = expression code="x*0.0075"(w1837) -> (w1835:dbl)
          }
        }
        n386 = Less?(x=w807, y="Low dP limit for Yoyo") -> (x < y?=w801:bool)
        n387 = Greater?(x=w807, y="High dP limit for Yoyo") -> (0:w792:bool)
        n388 = And(x=w792, y="Yoyo method while in\nAutomatic?") -> (x .and. y?=w791:bool)
        n389 = Select(t=TRUE, s="Start Yoyo", f=w791) -> (s? t:f=w795:bool)
        n390 = Select(t=w800, s=w795, f=w793) -> (s? t:f=w805:dbl)
        n391 = And(x=w801, y="Yoyo method while in\nAutomatic?") -> (x .and. y?=w790:bool)
        n392 = Select(t=w799, s=w790, f=w805) -> (s? t:f=w780:dbl)
        n393 = Negate(x=w780) -> ()  [unwired: 1 out]
        n394 = Negate(x=w780) -> (-x=w777:dbl)
        n395 = Add(x=w807, y=w780) -> (x+y=w815:dbl)
        n396 = Greater?(x=w815, y="delta (Dead band)\n(torr)") -> (0:w1452:bool)
        n397 = Less?(x=w815, y=w1808) -> (x < y?=w1451:bool)
        n398 = Greater Or Equal?(x=w815, y=w1808) -> (x >= y?=w1807:bool)
        n399 = Less?(x=w815, y=w1805) -> (x < y?=w1806:bool)
        n400 = Greater Or Equal?(x=w815, y=w1805) -> (x >= y?=w1804:bool)
        n401 = Less Or Equal?(x=w815, y="delta (Dead band)\n(torr)") -> (x <= y?=w1803:bool)
        n402 = And(x=w1807, y=w1806) -> (x .and. y?=w1450:bool)
        n403 = And(x=w1804, y=w1803) -> (x .and. y?=w1449:bool)
        n404 = Replace Array Subset(array=w1447, new element #1=w1452, index #1=0 ("index"), new element #2=w1451, index #2=1 ("index"), new element #3=w1450, index #3=2 ("index"), new element #4=w1449, index #4=3 ("index")) -> (w1448:bool[])
        n405 = Boolean To (0,1)(Boolean=w1448) -> (0, 1=w1801:i16[])
        n406 = Equal?(x="High dP limit for Yoyo", y=w777) -> (x = y?=w778:bool)
        n407 = Search 1D Array(1D array=w1801, element=1) -> (index of element=w1760:i32)  [unwired: 1 in]
        n408 = Equal?(x=w1778, y=w1760) -> (x = y?=w1800:bool)
        n409 = case shown="True" w1800 {
          tunnel: [0 ("index") w2078] -> w1761
          tunnel: w1798 -> [_ w2077]
          frame False {
          }
          frame True {
            n410 = Increment(x=w2077) -> (x+1=w2078:i32)
          }
        }
        n411 = Or(x=w791, y=w790) -> (x .or. y?=w776:bool)
        n412 = Or(x=w776, y=w772) -> (x .or. y?=w775:bool)
        n413 = case shown="True" w775 {
          tunnel: [0 ("element") w1825] -> w787
          tunnel: w771 -> [_ w1826]
          frame False {
          }
          frame True {
            n414 = Increment(x=w1826) -> (x+1=w1825:i32)
          }
        }
        n415 = In Range and Coerce(upper limit=10 ("element"), x=w787, lower limit=1) -> (In Range?=w782:bool)  [unwired: 1 out]
        n416 = Greater Or Equal?(x=w1761, y="Feed and Bleed\nDead Time (s)") -> (x >= y?=w1790:bool)
        n417 = Equal?(x=w1760, y=0 ("element")) -> (x = y?=w1797:bool)
        n418 = Equal?(x=w1760, y=1 ("element")) -> (x = y?=w1796:bool)
        n419 = Equal?(x=w1760, y=2 ("element")) -> (x = y?=w1793:bool)
        n420 = Equal?(x=w1760, y=3 ("element")) -> (x = y?=w1792:bool)
        n421 = Less?(x=w807, y=w1131) -> (x < y?=w1128:bool)
        n422 = Or(x=w1128, y=w1307) -> (x .or. y?=w1129:bool)
        n423 = Compound Arithmetic op=AND(w1129, w1107, w904) -> (w1127:bool)
        n424 = Absolute Value(x=w807) -> (abs(x)=w1168:dbl)
        n425 = And(x=w1790, y=w1797) -> (x .and. y?=w1789:bool)
        n426 = And(x=w1790, y=w1796) -> (x .and. y?=w1788:bool)
        n427 = And(x=w1790, y=w1793) -> (x .and. y?=w1787:bool)
        n428 = And(x=w1790, y=w1792) -> (x .and. y?=w1786:bool)
        n429 = Greater?(x=w1168, y="|dP| Maximum\n(torr)") -> (0:w932:bool)
        n430 = Not(x=w932) -> (.not. x?=w1133:bool)
        n431 = And(x=w1133, y=w1136) -> (x .and. y?=w1134:bool)
        n432 = case shown="False" "Manual Operation of HFE Valves?" {
          tunnel: w1127 -> [w2000 _]
          tunnel: [w2000 "Relief To \nWessington\n(HEV28/18)"] -> w1233
          tunnel: [w1999 "Vapor Fill\nValve \n(HEV17)"] -> w1236
          tunnel: w1134 -> [w1999 _]
          frame False {
          }
          frame True {
          }
        }
        n433 = Not(x=w932) -> (.not. x?=w933:bool)
        n434 = And(x="Manual Operation of Valves", y=w933) -> (x .and. y?=w935:bool)
        n435 = Absolute Value(x=w815) -> (abs(x)=w822:dbl)
        n436 = call-poly <vilib>:"PID.vi"("reinitialize? (F)"="Reinitialize\nXenon Heater PID", "output range"=w1019, "dt (s)"=w1372, "PID gains"="Xenon Heater PID Gains", "process variable"=w815, "setpoint"=0.0) -> ("output"=w848:dbl)  [unwired: 4 in, 1 out]
        n437 = Select(t=30.0 ("index"), s=w932, f=0.0 ("index")) -> (s? t:f=w1629:dbl)
        n438 = Select(t=36.0 ("index"), s=w1022, f=0.0 ("index")) -> (s? t:f=w1001:dbl)
        n439 = Greater Or Equal?(x="High", y="Low") -> (x >= y?=w1756:bool)
        n440 = Replace Array Subset(array=w1568, new element #1=w828, index #1=i16 50 ("precision (6)"), new element #2=w1420, index #2=i16 51 ("precision (6)"), new element #3=w1614, index #3=i16 52 ("precision (6)")) -> (w1567:dbl[])
        n441 = Replace Array Subset(array=w1567, new element #1=w1422, index #1=0 ("index"), new element #2=w1615, index #2=8 ("index"), new element #3=w1566, index #3=16 ("index"), new element #4=w1229, index #4=24 ("index"), new element #5=w1225, index #5=30 ("index"), new element #6=w1547, index #6=46 ("index"), new element #7=w1311, index #7=113 ("index"), new element #8=w1354, index #8=114 ("index"), new element #9=w900, index #9=120 ("index"), new element #10=w1275, index #10=135 ("index"), new element #11=w1278, index #11=139 ("index"), new element #12=w767, index #12=143 ("index"), new element #13=w1264, index #13=147 ("index"), new element #14=w1263, index #14=148 ("index"), new element #15=w1248, index #15=155 ("index"), new element #16=w1242, index #16=156 ("index"), new element #17=w1238, index #17=160 ("index"), new element #18=w1216, index #18=34 ("index"), new element #19=w1217, index #19=35 ("index"), new element #20=w1218, index #20=36 ("index")) -> (w852:dbl[])
        n442 = Replace Array Subset(array=w852, new element=w849, index=120) -> (w853:dbl[])
        n443 = Replace Array Subset(array=w853, new element #1=w1340, index #1=118 ("index"), new element #2=w1296, index #2=124 ("index"), new element #3=w1295, index #3=125 ("index"), new element #4=w1182, index #4=129 ("index"), new element #5=w1179, index #5=171 ("index")) -> (w1341:dbl[])
        n444 = Index Array(array=w852, index="Control TC") -> (element=w858:dbl)
        n445 = Replace Array Subset(array=w1465, new element #1=w858, index #1=0 ("index"), new element #2=w858, index #2=1 ("index"), new element #3=w858, index #3=2 ("index")) -> (w1466:dbl[])
        n446 = Sort 1D Array(array=w1466) -> (sorted array=w1784:dbl[])
        n447 = Index Array(array=w1784, index #1=2 ("index"), index #2=0 ("index")) -> (element #1=w1782:dbl, element #2=w1781:dbl)
        n448 = Subtract(x=w1782, y=w1781) -> (x-y=w1783:dbl)
        n449 = Greater?(x=w1783, y="Inner Cryostat \nTC Variation Max (K)") -> (0:w1785:bool)
        n450 = case shown="True" w1785 {
          tunnel: w1466 -> [w2070 _]
          tunnel: [w2069 w2073] -> w1777
          tunnel: w1784 -> [_ w2075]
          tunnel: [0.0 ("index") 5.0 ("index")] -> w1648
          frame False {
            n451 = Index Array(array=w2070, index=1) -> (element=w2069:dbl)
          }
          frame True {
            n452 = Index Array(array=w2075, index=1) -> (element=w2073:dbl)
          }
        }
        "Cryostat \nTemp. (K)" <- w1777
        n453 = Less?(x=w1777, y="Low") -> (x < y?=w1459:bool)
        n454 = Greater Or Equal?(x=w1777, y=w1758) -> (x >= y?=w1461:bool)
        n455 = Not Or(1:w1459, 2:w1461) -> (0:w1460:bool)
        n456 = Replace Array Subset(array=w1457, new element #1=w1461, index #1=0 ("index"), new element #2=w1460, index #2=1 ("index"), new element #3=w1459, index #3=2 ("index")) -> (w1458:bool[])
        n457 = Boolean To (0,1)(Boolean=w1458) -> (0, 1=w1776:i16[])
        n458 = Search 1D Array(1D array=w1776, element=1) -> (index of element=w1763:i32)  [unwired: 1 in]
        n459 = Equal?(x=w1763, y=w1769) -> (x = y?=w1774:bool)
        n460 = Equal?(x=0 ("element"), y=w1763) -> (x = y?=w1210:bool)
        n461 = Equal?(x=2 ("element"), y=w1763) -> (x = y?=w1768:bool)
        n462 = case shown="False" w1774 {
          tunnel: [0 ("index") w2067] -> w1762
          tunnel: w1773 -> [_ w2066]
          frame False {
          }
          frame True {
            n463 = Increment(x=w2066) -> (x+1=w2067:i32)
          }
        }
        n464 = Greater Or Equal?(x=w1762, y="Cryostat Fridge\nDead Time (s)") -> (x >= y?=w1772:bool)
        n465 = And(x=w1210, y=w1772) -> (x .and. y?=w1764:bool)
        n466 = And(x=w1768, y=w1772) -> (x .and. y?=w1767:bool)
        n467 = Less?(x=w1777, y="Inner Cryostat \nOvercool Temp (K)") -> (x < y?=w1766:bool)
        n468 = Not(x=w1766) -> (.not. x?=w1765:bool)
        n469 = Or(x=w1766, y=w1767) -> (x .or. y?=w1696:bool)
        n470 = And(x=w1765, y=w1764) -> (x .and. y?=w1211:bool)
        n471 = Select(t=32.0 ("index"), s=w1378, f=0.0 ("index")) -> (s? t:f=w1654:dbl)
        n472 = Select(t=66.0 ("index"), s=w1056, f=0.0 ("index")) -> (s? t:f=w1059:dbl)
        n473 = case shown="True" w1697 {
          tunnel: w1211 -> [_ w2060]
          tunnel: w1696 -> [_ w2059]
          frame False {
            w2058 = refnum<k21> "FieldPoint\\MPR2\\Relay Module 1\\Polycold 1 c0"  # FieldPoint IO Point
            w2057 = FALSE
            # "Close Valve"
            n474 = shared-variable "MPR1\\Real-Time Library.lvlib\\Polycold 1 Status"(w2057) -> ()  [unwired: 1 in, 1 out]
            n475 = call <vilib>:"FP Write (Boolean -IO).vi"("FieldPoint IO Point In"=w2058, "value"=w2057) -> ()  [unwired: 11 in, 3 out]
          }
          frame True {
            n476 = case shown="True" w2060 {
              frame False {
              }
              frame True {
                w2064 = refnum<k21> "FieldPoint\\MPR2\\Relay Module 1\\Polycold 1 c0"  # FieldPoint IO Point
                w2063 = TRUE
                # "Open Valve"
                n477 = shared-variable "MPR1\\Real-Time Library.lvlib\\Polycold 1 Status"(w2063) -> ()  [unwired: 1 in, 1 out]
                n478 = call <vilib>:"FP Write (Boolean -IO).vi"("FieldPoint IO Point In"=w2064, "value"=w2063) -> ()  [unwired: 11 in, 3 out]
              }
            }
            n479 = case shown="True" w2059 {
              frame False {
              }
              frame True {
                w2061 = refnum<k21> "FieldPoint\\MPR2\\Relay Module 1\\Polycold 1 c0"  # FieldPoint IO Point
                w2062 = FALSE
                # "Close Valve"
                n480 = shared-variable "MPR1\\Real-Time Library.lvlib\\Polycold 1 Status"(w2062) -> ()  [unwired: 1 in, 1 out]
                n481 = call <vilib>:"FP Write (Boolean -IO).vi"("FieldPoint IO Point In"=w2061, "value"=w2062) -> ()  [unwired: 11 in, 3 out]
              }
            }
          }
        }
        n482 = Subtract(x=w864, y=w1110) -> (x-y=w1098:dbl)
        n483 = Select(t="High", s=w1032, f="Low") -> (s? t:f=w1031:dbl)
        n484 = Select(t=1.0 ("index"), s=w1665, f=0.0 ("index")) -> (s? t:f=w1611:dbl)
        n485 = Select(t=22.0 ("index"), s=w1705, f=0.0 ("index")) -> (s? t:f=w1582:dbl)
        n486 = Select(t=4.0 ("index"), s=w1766, f=0.0 ("index")) -> (s? t:f=w1649:dbl)
        n487 = call <vilib>:"FP Write (Boolean -IO).vi"("FieldPoint IO Point In"=w1237, "value"=w1236) -> ()  [unwired: 11 in, 3 out]
        n488 = Select(t="High", s=w1756, f="Low") -> (s? t:f=w1757:dbl)
        n489 = Number To Fractional String(number=w828, width (-)=i16 5 ("precision (6)"), precision (6)=i16 2) -> (F-format string=w1442:string)  [unwired: 1 in]
        n490 = Select(t=27.0 ("index"), s=w1704, f=0.0 ("index")) -> (s? t:f=w1580:dbl)
        n491 = Greater?(x=w1146, y="Xe Vessel \nOverpressure (torr)") -> (0:w1819:bool)
        n492 = Select(t=67.0 ("index"), s=w1050, f=0.0 ("index")) -> (s? t:f=w1046:dbl)
        n493 = Greater?(x=w922, y="CC Shut-Off\nThreshold (Torr)") -> (0:w1700:bool)
        n494 = Greater?(x=w865, y="Inner Cryostat \nOverpress (torr)") -> (0:w1818:bool)
        n495 = Greater?(x=w1572, y="TC 1/2 Shut-Off\nThreshold (Torr)") -> (0:w1701:bool)
        n496 = Greater?(x=w1571, y="TC 1/2 Shut-Off\nThreshold (Torr)") -> (0:w1702:bool)
        n497 = Select(t=43.0 ("index"), s=w1112, f=0.0 ("index")) -> (s? t:f=w1362:dbl)
        n498 = property on="High" class="DigNum (strict)"("Value"=w1031) -> ()  [unwired: 2 in, 2 out]
        n499 = Greater?(x=w864, y="Cryostat High Liquid\nLevel Alarm (cm)") -> (0:w1043:bool)
        n500 = Select(t=23.0 ("index"), s=w1700, f=0.0 ("index")) -> (s? t:f=w1581:dbl)
        n501 = Replace Array Subset(array=w1555, new element #1=w1611, index #1=i16 0 ("precision (6)"), new element #2=w859, index #2=i16 79 ("precision (6)")) -> (w1554:dbl[])
        n502 = Multiply(x=w822, y="Prop Valve\nMult. Factor") -> (x*y=w1165:dbl)
        n503 = property on="High" class="DigNum (strict)"("Value"=w1757) -> ()  [unwired: 2 in, 2 out]
        n504 = Select(t=39.0 ("index"), s=w1819, f=0.0 ("index")) -> (s? t:f=w1623:dbl)
        n505 = Bundle("Low"=w1757, "Low"="Low") -> (w1755:cluster{"Low":dbl, "Low":dbl})  [unwired: 1 in]
        n506 = Select(t=40.0 ("index"), s=w1818, f=0.0 ("index")) -> (s? t:f=w1625:dbl)
        n507 = Replace Substring(2:w1438, 4:"VSET " ("string to write"), 5:w829) -> (1:w1444:string)  [unwired: 1 in, 1 out]
        n508 = Compound Arithmetic op=OR(w1700, w1682, w1702) -> (w1698:bool)
        n509 = Compound Arithmetic op=OR(w1700, w1316, w1701) -> (w1699:bool)
        n510 = call-poly <vilib>:"PID.vi"("reinitialize? (F)"="Reinitialize \nHFE Ballast Bottle\nHeater PID", "output range"=w1755, "dt (s)"=w1372, "PID gains"="HFE Ballast Bottle Heater PID Gains", "process variable"=w865, "setpoint"="Set Point") -> ("output"=w1379:dbl)  [unwired: 4 in, 1 out]
        n511 = Replace Substring(2:5 ("offset (0)"), 3:w1438, 4:w1442, 5:w1444) -> (1:w1443:string)  [unwired: 1 out]
        n512 = Select(t=68.0 ("index"), s=w1043, f=0.0 ("index")) -> (s? t:f=w1045:dbl)
        n513 = Replace Substring(2:2 ("offset (0)"), 3:10 ("offset (0)"), 4:"\r\n" ("string"), 5:w1443) -> ()  [unwired: 2 out]
        n514 = case shown="True" w1695 {
          tunnel: w1211 -> [_ w2052]
          tunnel: w1696 -> [_ w2051]
          frame False {
            w2050 = refnum<k21> "FieldPoint\\MPR2\\Relay Module 1\\Polycold 2 c1"  # FieldPoint IO Point
            w2049 = FALSE
            # "Close Valve"
            n515 = shared-variable "MPR1\\Real-Time Library.lvlib\\Polycold 2 Status"(w2049) -> ()  [unwired: 1 in, 1 out]
            n516 = call <vilib>:"FP Write (Boolean -IO).vi"("FieldPoint IO Point In"=w2050, "value"=w2049) -> ()  [unwired: 11 in, 3 out]
          }
          frame True {
            n517 = case shown="True" w2051 {
              frame False {
              }
              frame True {
                w2053 = refnum<k21> "FieldPoint\\MPR2\\Relay Module 1\\Polycold 2 c1"  # FieldPoint IO Point
                w2054 = FALSE
                # "Close Valve"
                n518 = shared-variable "MPR1\\Real-Time Library.lvlib\\Polycold 2 Status"(w2054) -> ()  [unwired: 1 in, 1 out]
                n519 = call <vilib>:"FP Write (Boolean -IO).vi"("FieldPoint IO Point In"=w2053, "value"=w2054) -> ()  [unwired: 11 in, 3 out]
              }
            }
            n520 = case shown="True" w2052 {
              frame False {
              }
              frame True {
                w2056 = refnum<k21> "FieldPoint\\MPR2\\Relay Module 1\\Polycold 2 c1"  # FieldPoint IO Point
                w2055 = TRUE
                # "Open Valve"
                n521 = shared-variable "MPR1\\Real-Time Library.lvlib\\Polycold 2 Status"(w2055) -> ()  [unwired: 1 in, 1 out]
                n522 = call <vilib>:"FP Write (Boolean -IO).vi"("FieldPoint IO Point In"=w2056, "value"=w2055) -> ()  [unwired: 11 in, 3 out]
              }
            }
          }
        }
        n523 = Unbundle("Recirc. Pump PID Gains") -> ("Proportional gain (Kc)"=w1011:dbl, "Integral time (Ti, min)"=w1010:dbl, "Derivative time (Td, min)"=w1009:dbl)
        n524 = Unbundle("Xenon Heater PID Gains") -> ("Proportional gain (Kc)"=w1006:dbl, "Integral time (Ti, min)"=w1005:dbl, "Derivative time (Td, min)"=w1004:dbl)
        n525 = Unbundle("Condenser PID Gains") -> ("Proportional gain (Kc)"=w960:dbl, "Integral time (Ti, min)"=w959:dbl, "Derivative time (Td, min)"=w958:dbl)
        n526 = Select(t=1.0 ("index"), s=w1107, f=0.0 ("index")) -> (s? t:f=w1106:dbl)
        n527 = Select(t=1.0 ("index"), s=w1103, f=0.0 ("index")) -> (s? t:f=w1102:dbl)
        n528 = In Range and Coerce(upper limit=2.2, x=w1165, lower limit=0.0) -> (coerced(x)=w826:dbl)  [unwired: 1 out]
        n529 = Not(x=w1375) -> (.not. x?=w1373:bool)
        n530 = expression code="x/2.2*0.075+0.02"(w826) -> (w808:dbl)
        n531 = Or(x=w1378, y=w1373) -> (x .or. y?=w1380:bool)
        n532 = call <vilib>:"FP Write (Boolean -IO).vi"("FieldPoint IO Point In"=w1044, "value"=w1043) -> ()  [unwired: 11 in, 3 out]
        n533 = Subtract(x=w807, y=w1155) -> (x-y=w1154:dbl)
        n534 = Replace Array Subset(array=w1341, new element #1="2 HFE \nManometers \nMax Var (torr)", index #1=60 ("index"), new element #2="2 Xe Manometers \nMax Var (torr)", index #2=61 ("index"), new element #3="Xe Vessel \nOverpressure (torr)", index #3=62 ("index"), new element #4="Inner Cryostat \nOverpress (torr)", index #4=63 ("index"), new element #5="Max diff between \ndP from gauge and\ndP from man. (torr)", index #5=64 ("index"), new element #6="|dP| Maximum\n(torr)", index #6=65 ("index"), new element #7="Feed and Bleed\nDead Time (s)", index #7=66 ("index"), new element #8="delta (Dead band)\n(torr)", index #8=67 ("index"), new element #9=w807, index #9=175 ("index"), new element #10="Prop Valve\nMult. Factor", index #10=176 ("index"), new element #11=w1154, index #11=177 ("index")) -> (w1156:dbl[])
        n535 = Select(t=0.0, s=w1380, f=w1379) -> (s? t:f=w1349:dbl)
        n536 = Not(x=w1698) -> (.not. x?=w1095:bool)
        n537 = Not(x=w1699) -> (.not. x?=w1097:bool)
        n538 = Number To Fractional String(number=w828, width (-)=i16 5 ("precision (6)"), precision (6)=i16 2) -> (F-format string=w830:string)  [unwired: 1 in]
        n539 = Less?(x=w766, y=300.0) -> (x < y?=w768:bool)
        n540 = Select(t=0.0 ("f"), s=w782, f="Yoyo\nMethod\nProp. Valves\nSetting") -> (s? t:f=w788:dbl)
        n541 = Select(t=w788, s="Yoyo method while in\nAutomatic?", f=w808) -> (s? t:f=w789:dbl)
        n542 = And(x=w768, y=w845) -> (x .and. y?=w770:bool)
        n543 = Multiply(x=w815, y="Prop Valve\nMult. Factor") -> (x*y=w819:dbl)
        n544 = Replace Substring(2:w834, 4:"VSET " ("string to write"), 5:w829) -> (1:w839:string)  [unwired: 1 in, 1 out]
        n545 = Select(t=w848, s=w770, f=0.0) -> (s? t:f=w847:dbl)
        n546 = Replace Substring(2:5 ("offset (0)"), 3:w834, 4:w830, 5:w839) -> (1:w838:string)  [unwired: 1 out]
        n547 = Replace Array Subset(array=w1470, new element #1="3 Condenser TC's \nVariation Max (K)", index #1=0 ("element"), new element #2="Condenser \nOvercool Temp (K)", index #2=1 ("element"), new element #3="High", index #3=2 ("element"), new element #4="Low", index #4=3 ("element"), new element #5="Set Point", index #5=4 ("element"), new element #6=w960, index #6=5 ("element"), new element #7=w959, index #7=6 ("element"), new element #8=w958, index #8=7 ("element")) -> (w957:dbl[])
        n548 = Replace Substring(2:10 ("offset (0)"), 3:10 ("offset (0)"), 4:";ISET 4\r\n" ("string"), 5:w838) -> (1:w827:string)  [unwired: 1 out]
        n549 = case shown="True" w1669 {
          tunnel: [w2028 w2036] -> w1678
          tunnel: w1681 -> [w2031 w2035]
          tunnel: w1680 -> [w2030 w2034]
          tunnel: [w2029 w2033] -> w1679
          tunnel: w827 -> [_ w2032]
          tunnel: w1668 -> [w2027 _]
          frame False {
            n550 = VISA Write(VISA resource name=w2031, write buffer=w2027, error in (no error)=w2030) -> (VISA resource name out=w2029:refnum<visa-resource-name>, error out=w2028:errorcluster)  [unwired: 1 out]
          }
          frame True {
            # "Write Voltage Value\nTo Cryostat Heater 1"
            n551 = VISA Write(VISA resource name=w2035, write buffer=w2032, error in (no error)=w2034) -> (VISA resource name out=w2033:refnum<visa-resource-name>, error out=w2036:errorcluster)  [unwired: 1 out]
          }
        }
        n552 = case shown="True" w1669 {
          tunnel: [w2019 w2026] -> w1670
          tunnel: w1673 -> [w2021 w2025]
          tunnel: w1672 -> [w2020 w2024]
          tunnel: [w2018 w2023] -> w1671
          tunnel: w827 -> [_ w2022]
          tunnel: w1668 -> [w2017 _]
          frame False {
            n553 = VISA Write(VISA resource name=w2021, write buffer=w2017, error in (no error)=w2020) -> (VISA resource name out=w2018:refnum<visa-resource-name>, error out=w2019:errorcluster)  [unwired: 1 out]
          }
          frame True {
            # "Write Voltage Value\nTo Cryostat Heater 2"
            n554 = VISA Write(VISA resource name=w2025, write buffer=w2022, error in (no error)=w2024) -> (VISA resource name out=w2023:refnum<visa-resource-name>, error out=w2026:errorcluster)  [unwired: 1 out]
          }
        }
        n555 = shared-variable "MPR1\\Real-Time Library.lvlib\\Data for MPR 2"(w957) -> ()  [unwired: 1 in, 1 out]
        n556 = In Range and Coerce(upper limit=2.2, x=w819, lower limit=0.0) -> (coerced(x)=w820:dbl)  [unwired: 1 out]
        n557 = case shown="False" w1694 {
          tunnel: w1211 -> [_ w2044]
          tunnel: w1696 -> [_ w2043]
          frame False {
            w2041 = refnum<k21> "FieldPoint\\MPR2\\Relay Module 1\\Polycold 3 c2"  # FieldPoint IO Point
            w2042 = FALSE
            # "Close Valve"
            n558 = shared-variable "MPR1\\Real-Time Library.lvlib\\Polycold 3 Status"(w2042) -> ()  [unwired: 1 in, 1 out]
            n559 = call <vilib>:"FP Write (Boolean -IO).vi"("FieldPoint IO Point In"=w2041, "value"=w2042) -> ()  [unwired: 11 in, 3 out]
          }
          frame True {
            n560 = case shown="True" w2043 {
              frame False {
              }
              frame True {
                w2046 = refnum<k21> "FieldPoint\\MPR2\\Relay Module 1\\Polycold 3 c2"  # FieldPoint IO Point
                w2045 = FALSE
                # "Close Valve"
                n561 = shared-variable "MPR1\\Real-Time Library.lvlib\\Polycold 3 Status"(w2045) -> ()  [unwired: 1 in, 1 out]
                n562 = call <vilib>:"FP Write (Boolean -IO).vi"("FieldPoint IO Point In"=w2046, "value"=w2045) -> ()  [unwired: 11 in, 3 out]
              }
            }
            n563 = case shown="True" w2044 {
              frame False {
              }
              frame True {
                w2048 = refnum<k21> "FieldPoint\\MPR2\\Relay Module 1\\Polycold 3 c2"  # FieldPoint IO Point
                w2047 = TRUE
                # "Open Valve"
                n564 = shared-variable "MPR1\\Real-Time Library.lvlib\\Polycold 3 Status"(w2047) -> ()  [unwired: 1 in, 1 out]
                n565 = call <vilib>:"FP Write (Boolean -IO).vi"("FieldPoint IO Point In"=w2048, "value"=w2047) -> ()  [unwired: 11 in, 3 out]
              }
            }
          }
        }
        n566 = expression code="x/2.2*0.075+0.02"(w820) -> (w814:dbl)
        n567 = case shown="False" w935 {
          tunnel: w1789 -> [w1879 _]
          tunnel: w1788 -> [w1878 _]
          tunnel: w1787 -> [w1877 _]
          tunnel: w1786 -> [w1876 _]
          tunnel: [w1857 w1961] -> w1196
          tunnel: [w1857 w1960] -> w1195
          tunnel: [w1874 w1959] -> w1194
          tunnel: [w1859 w1958] -> w1193
          tunnel: [w1856 w1957] -> w1192
          tunnel: [w1852 w1956] -> w1191
          tunnel: [w1868 w1948] -> w1153
          tunnel: [w1871 "V-X9"] -> w1151
          tunnel: w789 -> [w1875 _]
          tunnel: "V-X10" -> [_ w1986]
          tunnel: "V-X11" -> [_ w1985]
          tunnel: "V-X49" -> [_ w1984]
          tunnel: "V-X51" -> [_ w1982]
          tunnel: "V-X52" -> [_ w1981]
          tunnel: "V-X50" -> [_ w1983]
          tunnel: w843 -> [w1862 _]
          tunnel: w842 -> [w1860 _]
          tunnel: "Bleed 50?" -> [w1855 _]
          tunnel: w814 -> [_ w1944]
          tunnel: "Yoyo method while in\nAutomatic?" -> [w1854 _]
          tunnel: w778 -> [w1851 _]
          frame False {
            w1857 = FALSE
            w1863 = refnum<k21> "FieldPoint\\MPR1\\Digital Voltage Output Module 1\\V-X52 c6"  # FieldPoint IO Point
            w1864 = refnum<k21> "FieldPoint\\MPR1\\Digital Voltage Output Module 1\\V-X11 c4"  # FieldPoint IO Point
            w1865 = refnum<k21> "FieldPoint\\MPR1\\Digital Voltage Output Module 1\\V-X10 c5"  # FieldPoint IO Point
            # "Figure that\nshit out bitch!"
            n568 = flat-sequence {
              tunnel: w1879 -> [w1893]
              tunnel: w1878 -> [w1892]
              tunnel: w1877 -> [w1891]
              tunnel: w1876 -> [w1890]
              tunnel: w1875 -> [w1887]
              tunnel: [w1889] -> w1869
              tunnel: [w1888] -> w1870
              tunnel: [w1886] -> w1867
              tunnel: [w1885] -> w1866
              tunnel: w1862 -> [w1884]
              tunnel: [w1884] -> w1861
              tunnel: [w1939] -> w1874
              tunnel: [w1938] -> w1858
              tunnel: w1861 -> [w1937]
              frame #0 {
                n569 = case shown="True" w1890 {
                  tunnel: w1887 -> [_ w1897]
                  tunnel: [0.0 ("value") w1896] -> w1886
                  tunnel: w1884 -> [_ w1895]
                  frame False {
                  }
                  frame True {
                    n570 = call-poly <vilib>:"FP Read (Polymorphic).vi"("FieldPoint IO Point In"=refnum<k21> "FieldPoint\\MPR1\\Digital Voltage Output Module 1\\V-X49 c9" ("FieldPoint IO Point"), "Type"=TRUE) -> ("value"=w1898:bool)  [unwired: 10 in, 3 out]
                    n571 = case shown="True" w1898 {
                      tunnel: w1897 -> [w1901 _]
                      tunnel: [w1901 w1904] -> w1896
                      tunnel: w1895 -> [_ w1903]
                      frame False {
                        n572 = call <vilib>:"FP Write (Float -IO).vi"("FieldPoint IO Point In"=refnum<k21> "FieldPoint\\MPR2\\Analog Voltage Output Module 1\\V-X8 c0" ("FieldPoint IO Point"), "value"=w1901) -> ()  [unwired: 11 in, 3 out]
                      }
                      frame True {
                        w1904 = 0.0 ("value")
                        # "Bleed"
                        # "Feed"
                        n573 = call <vilib>:"FP Write (Boolean -IO).vi"("FieldPoint IO Point In"=refnum<k21> "FieldPoint\\MPR1\\Digital Voltage Output Module 1\\V-X49 c9" ("FieldPoint IO Point"), "value"=FALSE) -> ()  [unwired: 11 in, 3 out]
                        n574 = call <vilib>:"FP Write (Boolean -IO).vi"("FieldPoint IO Point In"=w1903, "value"=FALSE) -> ()  [unwired: 11 in, 3 out]
                        n575 = call <vilib>:"FP Write (Float -IO).vi"("FieldPoint IO Point In"=refnum<k21> "FieldPoint\\MPR2\\Analog Voltage Output Module 1\\V-X9 c1" ("FieldPoint IO Point"), "value"=w1904) -> ()  [unwired: 11 in, 3 out]
                      }
                    }
                  }
                }
                n576 = case shown="True" w1891 {
                  tunnel: w1887 -> [_ w1912]
                  tunnel: [0.0 ("value") w1911] -> w1885
                  tunnel: w1884 -> [_ w1910]
                  frame False {
                  }
                  frame True {
                    n577 = call-poly <vilib>:"FP Read (Polymorphic).vi"("FieldPoint IO Point In"=w1910, "Type"=TRUE) -> ("value"=w1913:bool)  [unwired: 10 in, 3 out]
                    n578 = case shown="True" w1913 {
                      tunnel: w1912 -> [w1915 _]
                      tunnel: [w1915 w1918] -> w1911
                      tunnel: w1910 -> [_ w1917]
                      frame False {
                        n579 = call <vilib>:"FP Write (Float -IO).vi"("FieldPoint IO Point In"=refnum<k21> "FieldPoint\\MPR2\\Analog Voltage Output Module 1\\V-X9 c1" ("FieldPoint IO Point"), "value"=w1915) -> ()  [unwired: 11 in, 3 out]
                      }
                      frame True {
                        w1918 = 0.0 ("value")
                        # "Bleed"
                        # "Feed"
                        n580 = call <vilib>:"FP Write (Boolean -IO).vi"("FieldPoint IO Point In"=refnum<k21> "FieldPoint\\MPR1\\Digital Voltage Output Module 1\\V-X49 c9" ("FieldPoint IO Point"), "value"=FALSE) -> ()  [unwired: 11 in, 3 out]
                        n581 = call <vilib>:"FP Write (Boolean -IO).vi"("FieldPoint IO Point In"=w1917, "value"=FALSE) -> ()  [unwired: 11 in, 3 out]
                        n582 = call <vilib>:"FP Write (Float -IO).vi"("FieldPoint IO Point In"=refnum<k21> "FieldPoint\\MPR2\\Analog Voltage Output Module 1\\V-X8 c0" ("FieldPoint IO Point"), "value"=w1918) -> ()  [unwired: 11 in, 3 out]
                      }
                    }
                  }
                }
                n583 = case shown="True" w1892 {
                  tunnel: w1887 -> [_ w1925]
                  tunnel: [0.0 w1925] -> w1888
                  tunnel: w1884 -> [_ w1924]
                  frame False {
                  }
                  frame True {
                    # "Bleed"
                    # "Feed"
                    n584 = call <vilib>:"FP Write (Boolean -IO).vi"("FieldPoint IO Point In"=refnum<k21> "FieldPoint\\MPR1\\Digital Voltage Output Module 1\\V-X49 c9" ("FieldPoint IO Point"), "value"=TRUE) -> ()  [unwired: 11 in, 3 out]
                    n585 = call <vilib>:"FP Write (Boolean -IO).vi"("FieldPoint IO Point In"=w1924, "value"=FALSE) -> ()  [unwired: 11 in, 3 out]
                    n586 = call <vilib>:"FP Write (Float -IO).vi"("FieldPoint IO Point In"=refnum<k21> "FieldPoint\\MPR2\\Analog Voltage Output Module 1\\V-X9 c1" ("FieldPoint IO Point"), "value"=w1925) -> ()  [unwired: 11 in, 3 out]
                  }
                }
                n587 = case shown="True" w1893 {
                  tunnel: w1887 -> [_ w1932]
                  tunnel: [0.0 w1932] -> w1889
                  tunnel: w1884 -> [_ w1931]
                  frame False {
                  }
                  frame True {
                    # "Bleed"
                    # "Feed"
                    n588 = call <vilib>:"FP Write (Boolean -IO).vi"("FieldPoint IO Point In"=refnum<k21> "FieldPoint\\MPR1\\Digital Voltage Output Module 1\\V-X49 c9" ("FieldPoint IO Point"), "value"=FALSE) -> ()  [unwired: 11 in, 3 out]
                    n589 = call <vilib>:"FP Write (Boolean -IO).vi"("FieldPoint IO Point In"=w1931, "value"=TRUE) -> ()  [unwired: 11 in, 3 out]
                    n590 = call <vilib>:"FP Write (Float -IO).vi"("FieldPoint IO Point In"=refnum<k21> "FieldPoint\\MPR2\\Analog Voltage Output Module 1\\V-X8 c0" ("FieldPoint IO Point"), "value"=w1932) -> ()  [unwired: 11 in, 3 out]
                  }
                }
              }
              frame #1 {
                n591 = call-poly <vilib>:"FP Read (Polymorphic).vi"("FieldPoint IO Point In"=refnum<k21> "FieldPoint\\MPR1\\Digital Voltage Output Module 1\\V-X49 c9" ("FieldPoint IO Point"), "Type"=TRUE) -> ("value"=w1939:bool)  [unwired: 10 in, 3 out]
                n592 = call-poly <vilib>:"FP Read (Polymorphic).vi"("FieldPoint IO Point In"=w1937, "Type"=TRUE) -> ("value"=w1938:bool)  [unwired: 10 in, 3 out]
              }
            }
            n593 = Select(t=w1851, s=w1854, f="VX52 real") -> (s? t:f=w1852:bool)
            n594 = call <vilib>:"FP Write (Boolean -IO).vi"("FieldPoint IO Point In"=w1860, "value"=w1857) -> ()  [unwired: 11 in, 3 out]
            n595 = call <vilib>:"FP Write (Boolean -IO).vi"("FieldPoint IO Point In"=w1865, "value"=w1857) -> ()  [unwired: 11 in, 3 out]
            n596 = call <vilib>:"FP Write (Boolean -IO).vi"("FieldPoint IO Point In"=w1863, "value"=w1852) -> ()  [unwired: 11 in, 3 out]
            n597 = call <vilib>:"FP Write (Boolean -IO).vi"("FieldPoint IO Point In"=w1864, "value"=w1857) -> ()  [unwired: 11 in, 3 out]
            n598 = Equal To 0?(x=w1870) -> (x = 0?=w1873:bool)
            n599 = Select(t=w1866, s=w1873, f=w1870) -> (s? t:f=w1871:dbl)
            n600 = Equal To 0?(x=w1869) -> (x = 0?=w1872:bool)
            n601 = Select(t=w1867, s=w1872, f=w1869) -> (s? t:f=w1868:dbl)
            n602 = case shown="False" w1855 {
              tunnel: [w1881 w1883] -> w1859
              tunnel: w1858 -> [w1880 w1883]
              tunnel: w1857 -> [w1881 w1882]
              tunnel: [w1880 w1882] -> w1856
              frame False {
              }
              frame True {
              }
            }
          }
          frame True {
            w1988 = refnum<k21> "FieldPoint\\MPR2\\Analog Voltage Output Module 1\\V-X9 c1"  # FieldPoint IO Point
            w1989 = refnum<k21> "FieldPoint\\MPR2\\Analog Voltage Output Module 1\\V-X8 c0"  # FieldPoint IO Point
            w1990 = refnum<k21> "FieldPoint\\MPR1\\Digital Voltage Output Module 1\\V-X52 c6"  # FieldPoint IO Point
            w1991 = refnum<k21> "FieldPoint\\MPR1\\Digital Voltage Output Module 1\\V-X51 c8"  # FieldPoint IO Point
            w1992 = refnum<k21> "FieldPoint\\MPR1\\Digital Voltage Output Module 1\\V-X50 c7"  # FieldPoint IO Point
            w1993 = refnum<k21> "FieldPoint\\MPR1\\Digital Voltage Output Module 1\\V-X49 c9"  # FieldPoint IO Point
            w1994 = refnum<k21> "FieldPoint\\MPR1\\Digital Voltage Output Module 1\\V-X11 c4"  # FieldPoint IO Point
            w1995 = refnum<k21> "FieldPoint\\MPR1\\Digital Voltage Output Module 1\\V-X10 c5"  # FieldPoint IO Point
            n603 = Search 1D Array(1D array="Valves to Open", element=11) -> (index of element=w1966:i32)  [unwired: 1 in]
            n604 = Search 1D Array(1D array="Valves to Open", element=52) -> (index of element=w1962:i32)  [unwired: 1 in]
            n605 = Search 1D Array(1D array="Valves to Open", element=50) -> (index of element=w1964:i32)  [unwired: 1 in]
            n606 = Search 1D Array(1D array="Valves to Open", element=10) -> (index of element=w1967:i32)  [unwired: 1 in]
            n607 = Search 1D Array(1D array="Valves to Open", element=51) -> (index of element=w1963:i32)  [unwired: 1 in]
            n608 = Search 1D Array(1D array="Valves to Open", element=49) -> (index of element=w1965:i32)  [unwired: 1 in]
            n609 = Not Equal?(x=w1967, y=-1 ("element")) -> (x != y?=w1955:bool)
            n610 = And(x=w1986, y=w1955) -> (x .and. y?=w1961:bool)
            n611 = call <vilib>:"FP Write (Boolean -IO).vi"("FieldPoint IO Point In"=w1995, "value"=w1961) -> ()  [unwired: 11 in, 3 out]
            n612 = Not Equal?(x=w1966, y=-1 ("element")) -> (x != y?=w1954:bool)
            n613 = And(x=w1954, y=w1985) -> (x .and. y?=w1960:bool)
            n614 = call <vilib>:"FP Write (Boolean -IO).vi"("FieldPoint IO Point In"=w1994, "value"=w1960) -> ()  [unwired: 11 in, 3 out]
            n615 = Not Equal?(x=w1965, y=-1 ("element")) -> (x != y?=w1953:bool)
            n616 = And(x=w1953, y=w1984) -> (x .and. y?=w1959:bool)
            n617 = call <vilib>:"FP Write (Boolean -IO).vi"("FieldPoint IO Point In"=w1993, "value"=w1959) -> ()  [unwired: 11 in, 3 out]
            n618 = Not Equal?(x=w1964, y=-1 ("element")) -> (x != y?=w1952:bool)
            n619 = And(x=w1983, y=w1952) -> (x .and. y?=w1958:bool)
            n620 = call <vilib>:"FP Write (Boolean -IO).vi"("FieldPoint IO Point In"=w1992, "value"=w1958) -> ()  [unwired: 11 in, 3 out]
            n621 = Not Equal?(x=w1963, y=-1 ("element")) -> (x != y?=w1951:bool)
            n622 = And(x=w1951, y=w1982) -> (x .and. y?=w1957:bool)
            n623 = call <vilib>:"FP Write (Boolean -IO).vi"("FieldPoint IO Point In"=w1991, "value"=w1957) -> ()  [unwired: 11 in, 3 out]
            n624 = Not Equal?(x=w1962, y=-1 ("element")) -> (x != y?=w1950:bool)
            n625 = And(x=w1950, y=w1981) -> (x .and. y?=w1956:bool)
            n626 = call <vilib>:"FP Write (Boolean -IO).vi"("FieldPoint IO Point In"=w1990, "value"=w1956) -> ()  [unwired: 11 in, 3 out]
            n627 = call <vilib>:"FP Write (Float -IO).vi"("FieldPoint IO Point In"=w1988, "value"="V-X9") -> ()  [unwired: 11 in, 3 out]
            n628 = Greater Than 0?(x=w1944) -> (x > 0?=w1946:bool)
            n629 = Select(t=w1944, s=w1946, f=0.0) -> (s? t:f=w1943:dbl)
            n630 = Select(t=w1943, s="Automatic Bleed\nWhen in Manual?", f="V-X8") -> (s? t:f=w1948:dbl)
            n631 = call <vilib>:"FP Write (Float -IO).vi"("FieldPoint IO Point In"=w1989, "value"=w1948) -> ()  [unwired: 11 in, 3 out]
          }
        }
        n632 = expression code="(x-0.02)/0.055"(w1153) -> (w1152:dbl)
        n633 = expression code="(x-0.02)/0.055"(w1151) -> (w1150:dbl)
        n634 = Replace Array Subset(array=w1156, new element #1="High", index #1=68 ("element"), new element #2="Low", index #2=69 ("element"), new element #3="Inner Cryostat \nTC Variation Max (K)", index #3=70 ("element"), new element #4="Inner Cryostat \nOvercool Temp (K)", index #4=71 ("element"), new element #5="Cryostat Fridge\nDead Time (s)", index #5=72 ("element"), new element #6=w1152, index #6=168 ("element"), new element #7=w1150, index #7=169 ("element")) -> (w1398:dbl[])
        n635 = Replace Array Subset(array=w1398, new element #1=w1405, index #1=105 ("element"), new element #2=w1400, index #2=107 ("element"), new element #3=w905, index #3=108 ("element"), new element #4=w809, index #4=110 ("element"), new element #5=w864, index #5=117 ("element"), new element #6=w1086, index #6=172 ("element"), new element #7=w1087, index #7=174 ("element")) -> (w1397:dbl[])
        n636 = Select(t=24.0 ("index"), s=w1701, f=0.0 ("index")) -> (s? t:f=w1577:dbl)
        n637 = Unbundle("HFE Ballast Bottle Heater PID Gains") -> ("Proportional gain (Kc)"=w1324:dbl, "Integral time (Ti, min)"=w1323:dbl, "Derivative time (Td, min)"=w1322:dbl)
        n638 = Select(t=41.0 ("index"), s=w1721, f=0.0 ("index")) -> (s? t:f=w1624:dbl)
        n639 = Select(t=26.0 ("index"), s=w1702, f=0.0 ("index")) -> (s? t:f=w1579:dbl)
        n640 = call <vilib>:"FP Write (Boolean -IO).vi"("FieldPoint IO Point In"=w1234, "value"=w1112) -> ()  [unwired: 11 in, 3 out]
        n641 = call <vilib>:"FP Write (Boolean -IO).vi"("FieldPoint IO Point In"=w1235, "value"=w1233) -> ()  [unwired: 11 in, 3 out]
        n642 = Select(t=57.0 ("index"), s=w935, f=0.0 ("index")) -> (s? t:f=w1116:dbl)
        n643 = Replace Array Subset(array=w1554, new element #1=w1627, index #1=36 ("index"), new element #2=w1626, index #2=37 ("index"), new element #3=w1623, index #3=38 ("index"), new element #4=w1625, index #4=39 ("index"), new element #5=w1624, index #5=40 ("index"), new element #6=w1116, index #6=56 ("index")) -> (w1553:dbl[])
        n644 = Replace Array Subset(array=w1553, new element #1=w1630, index #1=28 ("index"), new element #2=w1629, index #2=29 ("index"), new element #3=w1628, index #3=30 ("index"), new element #4=w874, index #4=82 ("index")) -> (w1552:dbl[])
        n645 = Replace Array Subset(array=w1552, new element #1=w1649, index #1=3 ("element"), new element #2=w1648) -> (w1551:dbl[])  [unwired: 1 in]
        n646 = Replace Array Subset(array=w1551, new element #1=w1654, index #1=31 ("index"), new element #2=w889, index #2=80 ("index"), new element #3=w1059, index #3=65 ("index"), new element #4=w1046, index #4=66 ("index"), new element #5=w1045, index #5=67 ("index"), new element #6="Manual Liquid\nLevel (cm)", index #6=81 ("index"), new element #7=w879, index #7=83 ("index")) -> (w1366:dbl[])
        n647 = Replace Array Subset(array=w1366, new element #1=w1365, index #1=41 ("index"), new element #2=w1362, index #2=42 ("index"), new element #3=w1346, index #3=43 ("index"), new element #4=w1345, index #4=44 ("index"), new element #5=w1120, index #5=55 ("index"), new element #6=w1106, index #6=57 ("index"), new element #7=w1102, index #7=58 ("index"), new element #8=w1099, index #8=59 ("index"), new element #9=w1098, index #9=60 ("index")) -> (w1113:dbl[])
        n648 = Replace Array Subset(array=w1113, new element #1=w955, index #1=33 ("index"), new element #2=w951, index #2=45 ("index"), new element #3=w1001, index #3=35 ("index")) -> (w1550:dbl[])
        n649 = Replace Array Subset(array=w1550, new element #1=w1597, index #1=17 ("index"), new element #2=w1595, index #2=18 ("index"), new element #3=w1596, index #3=19 ("index"), new element #4=w923, index #4=20 ("index"), new element #5=w1259, index #5=48 ("index"), new element #6=w1253, index #6=49 ("index"), new element #7=w1139, index #7=50 ("index"), new element #8=w1064, index #8=62 ("index"), new element #9=w1063, index #9=63 ("index"), new element #10=w1062, index #10=64 ("index"), new element #11=w918, index #11=73 ("index"), new element #12=w915, index #12=74 ("index"), new element #13=w912, index #13=75 ("index"), new element #14=w794, index #14=76 ("index"), new element #15=w794, index #15=77 ("index"), new element #16=w898, index #16=78 ("index")) -> (w1549:dbl[])
        n650 = Replace Array Subset(array=w1199, new element #1=w1196, index #1=45 ("element"), new element #2=w1195, index #2=46 ("element"), new element #3=w1194, index #3=47 ("element"), new element #4=w1193, index #4=48 ("element"), new element #5=w1192, index #5=49 ("element"), new element #6=w1191, index #6=50 ("element"), new element #7=w935, index #7=51 ("element")) -> (w1198:bool[])
        n651 = Replace Array Subset(array=w1198, new element #1="Reinitialize \nHFE Ballast Bottle\nHeater PID", index #1=12 ("element"), new element #2=FALSE ("new element/subarray"), index #2=13 ("element"), new element #3=w1375, index #3=18 ("element"), new element #4=w1112, index #4=19 ("element"), new element #5=w1233, index #5=20 ("element"), new element #6=w1236, index #6=21 ("element"), new element #7="Manual Operation of HFE Valves?", index #7=22 ("element"), new element #8=w1138, index #8=23 ("element")) -> (w1652:bool[])
        n652 = Replace Array Subset(array=w1652, new element #1="Reinitialize\nCondenser PID", index #1=14 ("element"), new element #2="Reinitialize\nRecirc. Pump PID", index #2=15 ("element"), new element #3="Reinitialize\nXenon Heater PID", index #3=16 ("element"), new element #4="Condenser \nin Use?", index #4=44 ("index")) -> (w1556:bool[])
        n653 = Replace Array Subset(array=w1556, new element #1="Manual Operation of Valves", index #1=17 ("length (rest)"), new element #2=w1570, index #2=0 ("length (rest)")) -> (w1419:bool[])
        n654 = Multiply(x=w1130, y=w1351) -> (x*y=w1352:dbl)
        n655 = Replace Array Subset(array=w1397, new element #1=0.0 ("new element/subarray"), index #1=73 ("element"), new element #2="Ballast Bottle\nOverpressure (psi)", index #2=74 ("element"), new element #3="High", index #3=75 ("element"), new element #4="Low", index #4=76 ("element"), new element #5="Set Point", index #5=77 ("element"), new element #6=w1324, index #6=78 ("element"), new element #7=w1323, index #7=79 ("element"), new element #8=w1322, index #8=80 ("element"), new element #9=w1130, index #9=111 ("element"), new element #10=w1349, index #10=112 ("element"), new element #11=w1351, index #11=115 ("element"), new element #12=w1352, index #12=116 ("element")) -> (w1306:dbl[])
        n656 = for {
          tunnel: w1419 -> [w2016] mode=indexing
          tunnel: [w2013] -> w1416 mode=indexing
          n657 = Select(t=1.0 ("index"), s=w2016, f=0.0 ("index")) -> (s? t:f=w2013:dbl)
        }
        n658 = Replace Array Subset(array=w1306, new element #1="HFE Relief to\nWessington \nThreshold (torr)", index #1=126 ("element"), new element #2="HFE Relief to\nAtmosphere\nThreshold (torr)", index #2=127 ("element"), new element #3="HFE Vapor Fill\nSet Point (torr)", index #3=128 ("element")) -> (w1305:dbl[])
        n659 = Replace Array Subset(array=w1305, new element #1="3 Condenser TC's \nVariation Max (K)", index #1=81 ("element"), new element #2="Condenser \nOvercool Temp (K)", index #2=82 ("element"), new element #3="High", index #3=83 ("element"), new element #4="Low", index #4=84 ("element"), new element #5="Set Point", index #5=85 ("element"), new element #6=w960, index #6=86 ("element"), new element #7=w959, index #7=87 ("element"), new element #8=w958, index #8=88 ("element"), new element #9="Max |dP|\nacross purifier", index #9=89 ("element"), new element #10="Recirc. Pump \nOutput \nHigh Limit", index #10=90 ("element"), new element #11="Recirc. Pump \nOutput \nLow Limit", index #11=91 ("element"), new element #12="dP across purifier\nset point value", index #12=92 ("element"), new element #13=w1011, index #13=93 ("element"), new element #14=w1010, index #14=94 ("element"), new element #15=w1009, index #15=95 ("element"), new element #16="Xenon Heater \nOutput \nHigh Limit", index #16=96 ("element"), new element #17="Xenon Heater \nOutput \nLow Limit", index #17=97 ("element"), new element #18=w1006, index #18=98 ("element"), new element #19=w1005, index #19=99 ("element"), new element #20=w1004, index #20=100 ("element")) -> (w1561:dbl[])
        n660 = Replace Array Subset(array=w1561, new element #1="CC Soft Threshold\nAlarm (Torr)", index #1=101 ("length (rest)"), new element #2="CC Shut-Off\nThreshold (Torr)", index #2=102 ("length (rest)"), new element #3="TC 1/2 Shut-Off\nThreshold (Torr)", index #3=103 ("length (rest)"), new element #4="TC 1/2 Soft Threshold\nAlarm (Torr)", index #4=104 ("length (rest)")) -> (w1560:dbl[])
        n661 = Multiply(x=w1037, y=w1069) -> (x*y=w1036:dbl)
        n662 = case shown="True" w1210 {
          tunnel: [w1997 w1998] -> w1208
          tunnel: w1209 -> [w1996 w1998]
          frame False {
            n663 = Increment(x=w1996) -> (x+1=w1997:dbl)
          }
          frame True {
          }
        }
        n664 = Number To Fractional String(number=w1349, width (-)=i16 5 ("precision (6)"), precision (6)=i16 2) -> (F-format string=w1384:string)  [unwired: 1 in]
        n665 = Number To Fractional String(number=w847, width (-)=i16 5 ("precision (6)"), precision (6)=i16 2) -> (F-format string=w1074:string)  [unwired: 1 in]
        n666 = Select(t="Valve 1 State", s="Manual Operation of Valves", f=w1097) -> (s? t:f=w1096:bool)
        n667 = Select(t="Valve 2 State", s="Manual Operation of Valves", f=w1095) -> (s? t:f=w1094:bool)
        n668 = call <vilib>:"FP Write (Boolean -IO).vi"("FieldPoint IO Point In"=w1214, "value"=w1094) -> ()  [unwired: 11 in, 3 out]
        n669 = call <vilib>:"FP Write (Boolean -IO).vi"("FieldPoint IO Point In"=w1215, "value"=w1096) -> ()  [unwired: 11 in, 3 out]
        n670 = Replace Array Subset(array=w1560, new element #1=w1576, index #1=39 ("length (rest)"), new element #2=w1149, index #2=40 ("length (rest)"), new element #3=w1574, index #3=41 ("length (rest)"), new element #4=w1148, index #4=42 ("length (rest)"), new element #5=w922, index #5=43 ("length (rest)"), new element #6=w1572, index #6=44 ("length (rest)"), new element #7=w1571, index #7=45 ("length (rest)"), new element #8=w1257, index #8=153 ("index"), new element #9=w1255, index #9=154 ("index"), new element #10=w1169, index #10=170 ("index")) -> (w1418:dbl[])
        n671 = Replace Substring(2:w1389, 4:"VSET " ("string to write"), 5:w829) -> (1:w1394:string)  [unwired: 1 in, 1 out]
        n672 = Replace Substring(2:w1079, 4:"VSET " ("string to write"), 5:w829) -> (1:w1084:string)  [unwired: 1 in, 1 out]
        n673 = Replace Substring(2:5 ("offset (0)"), 3:w1389, 4:w1384, 5:w1394) -> (1:w1393:string)  [unwired: 1 out]
        n674 = Select(t=62.0 ("index"), s="Manual Operation of Valves", f=0.0 ("index")) -> (s? t:f=w1089:dbl)
        n675 = Replace Substring(2:5 ("offset (0)"), 3:w1079, 4:w1074, 5:w1084) -> (1:w1083:string)  [unwired: 1 out]
        n676 = Replace Substring(2:10 ("offset (0)"), 3:10 ("offset (0)"), 4:";ISET 20\r\n" ("string"), 5:w1393) -> (1:w1387:string)  [unwired: 1 out]
        n677 = Replace Substring(2:10 ("offset (0)"), 3:10 ("offset (0)"), 4:";ISET 20\r\n" ("string"), 5:w1083) -> (1:w1077:string)  [unwired: 1 out]
        n678 = Replace Array Subset(array=w1418, new element=w1416, index=178 ("length (rest)")) -> (w1415:dbl[])
        n679 = Select(t=28.0 ("index"), s=w1663, f=0.0 ("index")) -> (s? t:f=w1548:dbl)
        n680 = Replace Array Subset(array=w1549, new element #1=w1582, index #1=21 ("length (rest)"), new element #2=w1581, index #2=22 ("length (rest)"), new element #3=w1577, index #3=23 ("length (rest)"), new element #4=w1578, index #4=24 ("length (rest)"), new element #5=w1579, index #5=25 ("length (rest)"), new element #6=w1580, index #6=26 ("length (rest)"), new element #7=w1548, index #7=27 ("length (rest)"), new element #8=w1089, index #8=61 ("length (rest)")) -> (w1034:dbl[])
        n681 = Replace Array Subset(array=w1034, new element #1=w847, index #1=68 ("length (rest)"), new element #2=w1037, index #2=69 ("length (rest)"), new element #3=w1069, index #3=70 ("length (rest)"), new element #4=w1036, index #4=71 ("length (rest)"), new element #5=w1035, index #5=72 ("length (rest)")) -> (w1033:dbl[])
        n682 = case shown="True" w863 {
          tunnel: [w2006 w2012] -> w1382
          tunnel: [w2007 w2011] -> w1383
          tunnel: w1387 -> [_ w2010]
          tunnel: "IOUT?;VOUT?\r\n" ("string to write") -> [w2005 _]
          tunnel: w1361 -> [w2004 w2009]
          tunnel: w1360 -> [w2003 w2008]
          frame False {
            n683 = VISA Write(VISA resource name=w2004, write buffer=w2005, error in (no error)=w2003) -> (VISA resource name out=w2007:refnum<visa-resource-name>, error out=w2006:errorcluster)  [unwired: 1 out]
          }
          frame True {
            # "Write Voltage Value\nTo Cryostat Heater 1"
            n684 = VISA Write(VISA resource name=w2009, write buffer=w2010, error in (no error)=w2008) -> (VISA resource name out=w2011:refnum<visa-resource-name>, error out=w2012:errorcluster)  [unwired: 1 out]
          }
        }
        n685 = Select(t=0.0, s="Restart all 3 Fridges until setpoint", f=w1208) -> (s? t:f=w1207:dbl)
        n686 = case shown="False" w1068 {
          tunnel: [w1844 w1850] -> w1072
          tunnel: [w1845 w1849] -> w1073
          tunnel: w1077 -> [_ w1848]
          tunnel: "IOUT?;VOUT?\r\n" ("string to write") -> [w1843 _]
          tunnel: w1071 -> [w1842 w1847]
          tunnel: w1070 -> [w1841 w1846]
          frame False {
            n687 = VISA Write(VISA resource name=w1842, write buffer=w1843, error in (no error)=w1841) -> (VISA resource name out=w1845:refnum<visa-resource-name>, error out=w1844:errorcluster)  [unwired: 1 out]
          }
          frame True {
            # "Write Voltage Value\nTo Cryostat Heater 1"
            n688 = VISA Write(VISA resource name=w1847, write buffer=w1848, error in (no error)=w1846) -> (VISA resource name out=w1849:refnum<visa-resource-name>, error out=w1850:errorcluster)  [unwired: 1 out]
          }
        }
        n689 = case shown="False" w1663 {
          tunnel: w1415 -> [w2038 w2040]
          tunnel: w1033 -> [w2037 w2039]
          frame False {
            # "Write to PC"
            n690 = shared-variable "MPR1\\Real-Time Library.lvlib\\Error Array for Monitor"(w2037) -> ()  [unwired: 1 in, 1 out]
            n691 = shared-variable "MPR1\\Real-Time Library.lvlib\\Data for Monitor"(w2038) -> ()  [unwired: 1 in, 1 out]
          }
          frame True {
            # "Write to Module"
            n692 = shared-variable "MPR1\\Real-Time Library.lvlib\\Error Array for Realtime"(w2039) -> ()  [unwired: 1 in, 1 out]
            n693 = shared-variable "MPR1\\Real-Time Library.lvlib\\Data for Realtime"(w2040) -> ()  [unwired: 1 in, 1 out]
          }
        }
      }
    }
    n694 = node-c288() -> ()  [unwired: 1 in, 1 out]
    "Loop Index" <- w237
  }
  n695 = node-c288(w108) -> (w112:T4)  [unwired: 3 in]
  n696 = timed-loop {
    shift-right: [w2115] -> _
    shift-left: TRUE -> [w2116]
    shift-right: [w2114] -> _
    shift-left: _ -> [w2113]
    shift-right: [w2110] -> _
    shift-left: _ -> [w2109]
    shift-right: [w2112] -> _
    shift-left: _ -> [w2111]
    timing: w112 -> [_]
    timing-out: [_] -> w111
    tunnel: "Folder to Store Data if Monitoring Program fails" -> [w2108]
    shift-right: [w2100] -> _
    shift-left: _ -> [w2104]
    shift-right: [w2091] -> _
    shift-left: _ -> [w2106]
    tunnel: w108 -> [w2098]
    i -> [w2107]
    stop <- _ stop-if-true
    w2091 = 6000 ("y")
    # "Have at\nleast 5\nfree Mb"
    n697 = node-c288() -> ()  [unwired: 1 in, 1 out]
    n698 = Get Volume Info(11:path "c:/" ("path")) -> (2:w2095:i64)  [unwired: 1 in, 5 out]
    n699 = Greater?(x=w2095, y=5000000.0) -> (0:w2093:bool)
    n700 = case shown="True" FALSE ("Boolean") {
      tunnel: w2116 -> [_ w2158]
      tunnel: [TRUE w2157] -> w2115
      tunnel: [w2120 w2156] -> w2114
      tunnel: w2113 -> [_ w2155]
      tunnel: [w2120 w2154] -> w2112
      tunnel: w2111 -> [_ w2153]
      tunnel: [w2120 w2152] -> w2110
      tunnel: w2109 -> [_ w2151]
      tunnel: w2108 -> [_ w2124]
      tunnel: w2107 -> [_ w2123]
      frame False {
        w2120 = i64 0
      }
      frame True {
        # "Large Data Array"
        n701 = shared-variable "MPR1\\Real-Time Library.lvlib\\Data for Realtime"() -> (w2122:dbl[])  [unwired: 1 in, 1 out]
        n702 = Equal To 0?(x=w2122) -> (x = 0?=w2142:bool[])
        n703 = Get Date/Time In Seconds() -> (seconds since 1Jan1904=w2137:timestamp)
        n704 = To Quad Integer(1:w2137) -> (0:w2133:i64)
        n705 = To Double Precision Float(number=w2137) -> (double precision float=w2141:dbl)
        n706 = And Array Elements(Boolean array=w2142) -> (logical AND=w2157:bool)
        n707 = Insert Into Array(array=w2122, index=0, new element=w2141) -> (w2125:dbl[])
        n708 = Or(x=w2157, y=w2158) -> (x .or. y?=w2140:bool)
        n709 = Not(x=w2157) -> (.not. x?=w2126:bool)
        n710 = Select(t=0, s=w2140, f=w2123) -> (s? t:f=w2139:i32)
        n711 = Quotient & Remainder(x=w2139, y=3600) -> (x-y*floor(x/y)=w2136:i32)  [unwired: 1 out]
        n712 = Equal To 0?(x=w2136) -> (x = 0?=w2132:bool)
        n713 = Select(t=w2133, s=w2132, f=w2155) -> (s? t:f=w2156:i64)
        n714 = And(x=w2126, y=w2132) -> (x .and. y?=w2129:bool)
        n715 = case shown="True" w2129 {
          tunnel: w2156 -> [_ w2187]
          tunnel: w2125 -> [_ w2185]
          tunnel: w2124 -> [_ w2182]
          frame False {
          }
          frame True {
            n716 = Array Size(array=w2185) -> (size(s)=w2186:i32)
            n717 = Concatenate Strings(w2182, "_1_index") -> (w2179:string)
            n718 = String To Path(string=w2179) -> (path=w2180:path)
            n719 = Build Array(w2186, w2187) -> (w2188:i64[])
            n720 = call-poly <vilib>:"Write To Spreadsheet File.vi"("format (%d)"="%.0f" ("format (%.3f)"), "append to file? (new file:F)"=TRUE, "1D data"=w2188, "file path (dialog if empty)"=w2180) -> ()  [unwired: 4 in, 1 out]
          }
        }
        n721 = Quotient & Remainder(x=w2139, y=60) -> (x-y*floor(x/y)=w2146:i32)  [unwired: 1 out]
        n722 = Quotient & Remainder(x=w2139, y=216000) -> (x-y*floor(x/y)=w2135:i32)  [unwired: 1 out]
        n723 = Equal To 0?(x=w2135) -> (x = 0?=w2131:bool)
        n724 = Select(t=w2133, s=w2131, f=w2153) -> (s? t:f=w2154:i64)
        n725 = And(x=w2131, y=w2126) -> (x .and. y?=w2128:bool)
        n726 = case shown="True" w2128 {
          tunnel: w2154 -> [_ w2177]
          tunnel: w2125 -> [_ w2175]
          tunnel: w2124 -> [_ w2172]
          frame False {
          }
          frame True {
            n727 = Array Size(array=w2175) -> (size(s)=w2176:i32)
            n728 = Build Array(w2176, w2177) -> (w2178:i64[])
            n729 = Concatenate Strings(w2172, "_60_index") -> (w2169:string)
            n730 = String To Path(string=w2169) -> (path=w2170:path)
            n731 = call-poly <vilib>:"Write To Spreadsheet File.vi"("format (%d)"="%.0f" ("format (%.3f)"), "append to file? (new file:F)"=TRUE, "1D data"=w2178, "file path (dialog if empty)"=w2170) -> ()  [unwired: 4 in, 1 out]
          }
        }
        n732 = Quotient & Remainder(x=w2139, y=3600) -> (x-y*floor(x/y)=w2144:i32)  [unwired: 1 out]
        n733 = Quotient & Remainder(x=w2139, y=12960000) -> (x-y*floor(x/y)=w2134:i32)  [unwired: 1 out]
        n734 = Equal To 0?(x=w2134) -> (x = 0?=w2130:bool)
        n735 = Select(t=w2133, s=w2130, f=w2151) -> (s? t:f=w2152:i64)
        n736 = case shown="True" w2126 {
          tunnel: w2154 -> [_ w2195]
          tunnel: w2146 -> [_ w2194]
          tunnel: w2144 -> [_ w2193]
          tunnel: w2124 -> [_ w2192]
          tunnel: w2152 -> [_ w2191]
          tunnel: w2125 -> [_ w2190]
          tunnel: w2156 -> [_ w2189]
          frame False {
          }
          frame True {
            # "Record Every 3600th Point"
            # "Record Every 60th Point"
            # "Record Every Point"
            n737 = flat-sequence {
              tunnel: w2192 -> [w2197]
              tunnel: w2190 -> [w2201]
              tunnel: w2189 -> [w2198]
              tunnel: w2195 -> [w2209]
              tunnel: w2194 -> [w2207]
              tunnel: w2192 -> [w2206]
              tunnel: w2190 -> [w2205]
              tunnel: w2193 -> [w2221]
              tunnel: w2192 -> [w2220]
              tunnel: w2190 -> [w2219]
              tunnel: w2191 -> [w2218]
              frame #0 {
                n738 = Number To Decimal String(number=w2198, width (-)=i16 10) -> (decimal integer string=w2202:string)
                n739 = Concatenate Strings(w2197, "_1_", w2202) -> (w2204:string)
                n740 = String To Path(string=w2204) -> (path=w2203:path)
                n741 = call "Write To DBL File.vi"("append to file? (new file:F)"=TRUE, "1D array"=w2201, "file path (dialog if empty)"=w2203) -> ()  [unwired: 4 in, 1 out]
              }
              frame #1 {
                n742 = Equal To 0?(x=w2207) -> (x = 0?=w2208:bool)
                n743 = case shown="True" w2208 {
                  tunnel: w2209 -> [_ w2214]
                  tunnel: w2206 -> [_ w2212]
                  tunnel: w2205 -> [_ w2211]
                  frame False {
                  }
                  frame True {
                    n744 = Number To Decimal String(number=w2214) -> (decimal integer string=w2217:string)  [unwired: 1 in]
                    n745 = Concatenate Strings(w2212, "_60_", w2217) -> (w2215:string)
                    n746 = String To Path(string=w2215) -> (path=w2213:path)
                    n747 = call "Write To DBL File.vi"("append to file? (new file:F)"=TRUE, "1D array"=w2211, "file path (dialog if empty)"=w2213) -> ()  [unwired: 4 in, 1 out]
                  }
                }
              }
              frame #2 {
                n748 = Equal To 0?(x=w2221) -> (x = 0?=w2222:bool)
                n749 = case shown="True" w2222 {
                  tunnel: w2218 -> [_ w2227]
                  tunnel: w2220 -> [_ w2225]
                  tunnel: w2219 -> [_ w2224]
                  frame False {
                  }
                  frame True {
                    n750 = Number To Decimal String(number=w2227) -> (decimal integer string=w2230:string)  [unwired: 1 in]
                    n751 = Concatenate Strings(w2225, "_3600_", w2230) -> (w2228:string)
                    n752 = String To Path(string=w2228) -> (path=w2226:path)
                    n753 = call "Write To DBL File.vi"("append to file? (new file:F)"=TRUE, "1D array"=w2224, "file path (dialog if empty)"=w2226) -> ()  [unwired: 4 in, 1 out]
                  }
                }
              }
            }
          }
        }
        n754 = And(x=w2130, y=w2126) -> (x .and. y?=w2127:bool)
        n755 = case shown="True" w2127 {
          tunnel: w2152 -> [_ w2167]
          tunnel: w2125 -> [_ w2165]
          tunnel: w2124 -> [_ w2162]
          frame False {
          }
          frame True {
            n756 = Array Size(array=w2165) -> (size(s)=w2166:i32)
            n757 = Concatenate Strings(w2162, "_3600_index") -> (w2159:string)
            n758 = String To Path(string=w2159) -> (path=w2160:path)
            n759 = Build Array(w2166, w2167) -> (w2168:i64[])
            n760 = call-poly <vilib>:"Write To Spreadsheet File.vi"("format (%d)"="%.0f" ("format (%.3f)"), "append to file? (new file:F)"=TRUE, "1D data"=w2168, "file path (dialog if empty)"=w2160) -> ()  [unwired: 4 in, 1 out]
          }
        }
      }
    }
    n761 = Equal?(x=w2106, y=w2091) -> (x = y?=w2105:bool)
    n762 = case shown="True" w2105 {
      tunnel: w2104 -> [_ w2119]
      tunnel: [0 ("t") w2118] -> w2100
      frame False {
      }
      frame True {
        n763 = Increment(x=w2119) -> (x+1=w2118:i32)
      }
    }
    n764 = Divide(x=6000 ("y"), y=w2098) -> (x/y=w2103:dbl)
    n765 = Greater?(x=w2100, y=w2103) -> (0:w2094:bool)
    n766 = And(x=w2093, y=w2094) -> ()  [unwired: 1 out]
    n767 = Divide(x=3000 ("y"), y=w2098) -> (x/y=w2101:dbl)
    n768 = Greater?(x=w2100, y=w2101) -> ()  [unwired: 1 out]
    n769 = node-c288() -> ()  [unwired: 1 in, 1 out]
  }
  n770 = node-c288(w111) -> ()  [unwired: 1 out]
  n771 = node-c288(w115) -> ()  [unwired: 1 out]
  n772 = VISA Close(VISA resource name=w102, error in (no error)=w101) -> (error out=w103:errorcluster)
  n773 = VISA Close(VISA resource name=w96, error in (no error)=w95) -> (error out=w98:errorcluster)
  n774 = VISA Close(VISA resource name=w63, error in (no error)=w62) -> (error out=w64:errorcluster)
  n775 = call <vilib>:"Simple Error Handler.vi"("type of dialog (OK msg:1)"=w104, "error in (no error)"=w103) -> ()  [unwired: 3 in, 5 out]
  n776 = call <vilib>:"Simple Error Handler.vi"("type of dialog (OK msg:1)"=w97, "error in (no error)"=w98) -> ()  [unwired: 3 in, 5 out]
  n777 = VISA Close(VISA resource name=w31, error in (no error)=w30) -> (error out=w34:errorcluster)
  n778 = VISA Close(VISA resource name=w5, error in (no error)=w4) -> (error out=w7:errorcluster)
  n779 = VISA Close(VISA resource name=w118, error in (no error)=w117) -> (error out=w119:errorcluster)
  n780 = VISA Close(VISA resource name=w16, error in (no error)=w15) -> (error out=w17:errorcluster)
  n781 = VISA Close(VISA resource name=w45, error in (no error)=w44) -> (error out=w47:errorcluster)
  n782 = call <vilib>:"Simple Error Handler.vi"("type of dialog (OK msg:1)"=w65, "error in (no error)"=w64) -> ()  [unwired: 3 in, 5 out]
  n783 = call <vilib>:"Simple Error Handler.vi"("type of dialog (OK msg:1)"=w35, "error in (no error)"=w34) -> ()  [unwired: 3 in, 5 out]
  n784 = call <vilib>:"Simple Error Handler.vi"("type of dialog (OK msg:1)"=w6, "error in (no error)"=w7) -> ()  [unwired: 3 in, 5 out]
  n785 = call <vilib>:"Simple Error Handler.vi"("type of dialog (OK msg:1)"=w120, "error in (no error)"=w119) -> ()  [unwired: 3 in, 5 out]
  n786 = call <vilib>:"Simple Error Handler.vi"("type of dialog (OK msg:1)"=w18, "error in (no error)"=w17) -> ()  [unwired: 3 in, 5 out]
  n787 = call <vilib>:"Simple Error Handler.vi"("type of dialog (OK msg:1)"=w46, "error in (no error)"=w47) -> ()  [unwired: 3 in, 5 out]
